vi "Interfaz grafica - corriente.vi"() -> ()   [LabVIEW 2024]
uses:
  160620 Optotune Lens Driver 4 Labview package/Hello Optotune Lens (30.06.2015)/Calibration.ctl
  <vilib>/DAQmx/read.llb/DAQmx Read (Analog 1D Wfm NChan NSamp).vi
  <vilib>/Analysis/2dsp.llb/Decimate (single shot, DBL).vi
  <vilib>/Utility/file.llb/Read Delimited Spreadsheet (string).vi
  <vilib>/Instr/_visa.llb/VISA Configure Serial Port (Instr).vi
  <vilib>/DAQmx/create/channels.llb/DAQmx Create Channel (AI-Voltage-Basic).vi
  <vilib>/DAQmx/configure/timing.llb/DAQmx Timing (Sample Clock).vi
  <vilib>/DAQmx/miscellaneous.llb/DAQmx Fill In Error Info.vi
  <vilib>/Waveform/WDTOps.llb/WDT Index Channel DBL.vi
  <vilib>/Analysis/2dsp.llb/Decimate (continuous, DBL).vi
  <vilib>/Utility/file.llb/Write Delimited Spreadsheet (string).vi
  <vilib>/Waveform/WDTOps.llb/WDT Get Waveform Time Array DBL.vi
  <vilib>/Analysis/NI_AALPro.lvlib
panel:
  out "Array 4":string[](array[string])
  out "Array 3":string[](array[string])
  out "Array 2":string[](array[string])
  out "Array":string[](array[string])
  out "Nombre 2":string
  in  "Restablecer Iniciales":bool
  in  "Incremento":dbl=0.1 format="%#_13g"
  out "Potencia derecho":dbl
  out "error out 4":errorcluster
  out "error out 3":errorcluster
  out "error out 2":errorcluster
  in  "Tab Control 3":enum32{"WL", "Video"}(tab)
  out "Waveform length":dbl[][](graph)
  in  "Minimo escala Y":dbl format="%#_13g"
  in  "Maximo escala Y":dbl format="%#_13g"
  in  "Escala autom. Y":u8=1
  in  "Escala autom. X":u8=1
  in  "Maximo escala X":dbl
  in  "Minimo escala X":dbl
  out "Image Out":T1(plugin-control)
  in  "Frame Rate":u32=30
  in  "Modo de video":u16(ring)=21 items=["160x90 I420 30 fps", "160x90 MJPG 30 fps", "160x90 RGB24 30 fps", "160x120 I420 30 fps", "160x120 MJPG 30 fps", "160x120 RGB24 30 fps", "176x144 I420 30 fps", "176x144 MJPG 30 fps", "176x144 RGB24 30 fps", "320x180 I420 30 fps", "320x180 MJPG 30 fps", "320x180 RGB24 30 fps", "320x240  I420 30 fps", "320x240 MJPG 30 fps", "320x240 RGB24 30 fps", "352x288 I420 30 fps", "352x288 MJPG 30 fps", "352x288 RGB24 30 fps", "432x240 I420 30 fps", "432x240 MJPG 30 fps", "432x240 RGB24 30 fps", "640x360 I420 30 fps", "640x360 MJPG 30 fps", "640x360 RGB24 30 fps", "640x480 I420 30 fps", "640x480 MJPG 30 fps", "640x480 RGB24 30 fps", "800x448 I420 30 fps", "800x448 MJPG 30 fps", "800x448 RGB24 30 fps", "800x600 I420 30 fps", "800x600 MJPG 30 fps", "800x600 RGB24 30 fps", "864x480 I420 30 fps", "864x480 MJPG 30 fps", "864x480 RGB24 30 fps", "960x720 I420 30 fps", "960x720 MJPG 30 fps", "960x720 RGB24 30 fps", "1024x576 I420 30 fps", "1024x576 MJPG 30 fps", "1024x576 RGB24 30 fps", "1280x720 I420 30 fps", "1280x720 MJPG 30 fps", "1280x720 RGB24 30 fps", "1600x896 I420 30 fps", "1600x896 MJPG 30 fps", "1600x896 RGB24 30 fps", "1920x1080 I420 5 fps", "1920x1080 MJPG 30 fps", "1920x1080 RGB24 5 fps", "2304x1296 I420 2 fps", "2304x1296 RGB24 2 fps", "2304x1536 I420 2 fps", "2304x1536 RGB24 2 fps"]
  in  "Carpeta archivo":string="C:\\Users\\TGM1603\\Documents\\LabVIEW Data\\Experimentos electrodos\\VideosExperimentos"
  in  "Calidad":u32=1000
  out "VISA resource name out":string
  in  "Tab Control 2":T2(tab)
  in  "DAQmx Physical Channel":tag
  in  "Frecuencia muestreo":i32=20000
  in  "tamaño buffer":i32=1000
  in  "factor decimacion":i32=20
  in  "Ganancia":u16(ring) items=["0.2"=51455, "1"=33023, "10"=49407, "20"=41215, "30"=57599, "40"=37119, "60"=53503, "80"=45311, "120"=61695, "157"=35071, ""=0]
  in  "Potencia inicial lente derecho":dbl(slide) scale=-3.0..3.0
  in  "Potencia inicial lente izquierdo":dbl(slide) scale=-3.0..3.0
  in  "VISA resource name":string="COM11"
  in  "VISA resource name 2":string="COM10"
  out "DPT INICIALES D":dbl
  out "DPT INICIALES I":dbl
  out "Potencia izquierdo":dbl
  in  "error in (no error) 5":errorcluster
  in  "error in (no error) 4":errorcluster
  in  "error in (no error) 3":errorcluster
  in  "error in (no error) 2":errorcluster
  in  "Calibration 4":T3={"Max Current A"=293.0, "Max Current B"=293.0, "UCL A"=300.0, "UCL B"=300.0, "LCL A"=0.0, "LCL B"=0.0} {"Max Current A" format="%#_g mA"; "Max Current B" format="%#_g mA"; "UCL A" format="%#_g mA"; "LCL A" format="%#_g mA"; "UCL B" format="%#_g mA"; "LCL B" format="%#_g mA"}
  out "ID 2":u16
  out "VISA resource name out 2":string
  out "Calibration 3":T3 {"Max Current A" format="%#_g mA"; "Max Current B" format="%#_g mA"; "UCL A" format="%#_g mA"; "LCL A" format="%#_g mA"; "UCL B" format="%#_g mA"; "LCL B" format="%#_g mA"}
  out "OK 2":bool
  out "Data 2":string
  out "Command to Port 2":string
  in  "Cola tipo 2":dbl[](array[numeric])
  out "Distancia":u32
  in  "Tamaño ventana WL":i32=60
  in  "Limite inferior WL":dbl=25.0 format="%#_13g"
  in  "Limite superior WL":dbl=50.0
  out "number":u32
  in  "Calibration":T3={"Max Current A"=293.0, "Max Current B"=293.0, "UCL A"=300.0, "UCL B"=300.0, "LCL A"=0.0, "LCL B"=0.0} {"Max Current A" format="%#_g mA"; "Max Current B" format="%#_g mA"; "UCL A" format="%#_g mA"; "LCL A" format="%#_g mA"; "UCL B" format="%#_g mA"; "LCL B" format="%#_g mA"}
  out "ID":u16
  out "Calibration 2":T3 {"Max Current A" format="%#_g mA"; "Max Current B" format="%#_g mA"; "UCL A" format="%#_g mA"; "LCL A" format="%#_g mA"; "UCL B" format="%#_g mA"; "LCL B" format="%#_g mA"}
  out "OK":bool
  out "Data":string
  out "Command to Port":string
  in  "DPT dif.":dbl
  out "error out":errorcluster
  in  "error in (no error)":errorcluster
  in  "WL":dbl
  in  "Cola tipo":dbl[](array[numeric])
  out "T button?":bool
  in  "Elegir menu Exp":bool
  in  "Elegir menu":bool
  out "path":path
  in  "Iniciar experimento":bool
  in  "Parar adquisicion":bool
  out "Enfermedad visual":string
  out "Edad":string
  out "Nombre":string
  out "Cedula":string
  in  "Carpeta":path=path "C:/Users/TGM1603/Documents/LabVIEW Data/Experimentos electrodos"
  in  "?":bool
  in  "Menu Principal":u16(ring) items=["Visualizacion general ", "Llevar a cabo un experimento", "Ajustar potencia inicial lentes"]
  in  "Menu experimentos":u16(ring) items=["Experimento 1", "Experimento 2", "Experimento 3", "Experimento 4"]
  in  "Tab Control":enum32{"Señal EMG", "Potencia y distancia"}(tab)
  out "Senal EMG":waveform(dbl)[](graph)
  in  "Escala automatica Y":u8
  in  "Escala automatica X":u8=1
  in  "X Scale.Range:Increment":dbl
  in  "X Scale.Range:Minimum":dbl
  in  "X Scale.Range:Maximum":dbl
  in  "Y Scale.Range:Minimum":dbl=-5.0
  in  "Y Scale.Range:Maximum":dbl=5.0
  in  "Escala Y min":dbl
  in  "Escala Y max":dbl
  in  "Auto scale Y":u8=1
  in  "Escala X max":dbl
  in  "Escala X min":dbl
  out "Potencia optica y distancia":dbl[][](graph)
  in  "Auto scale X":u8=1
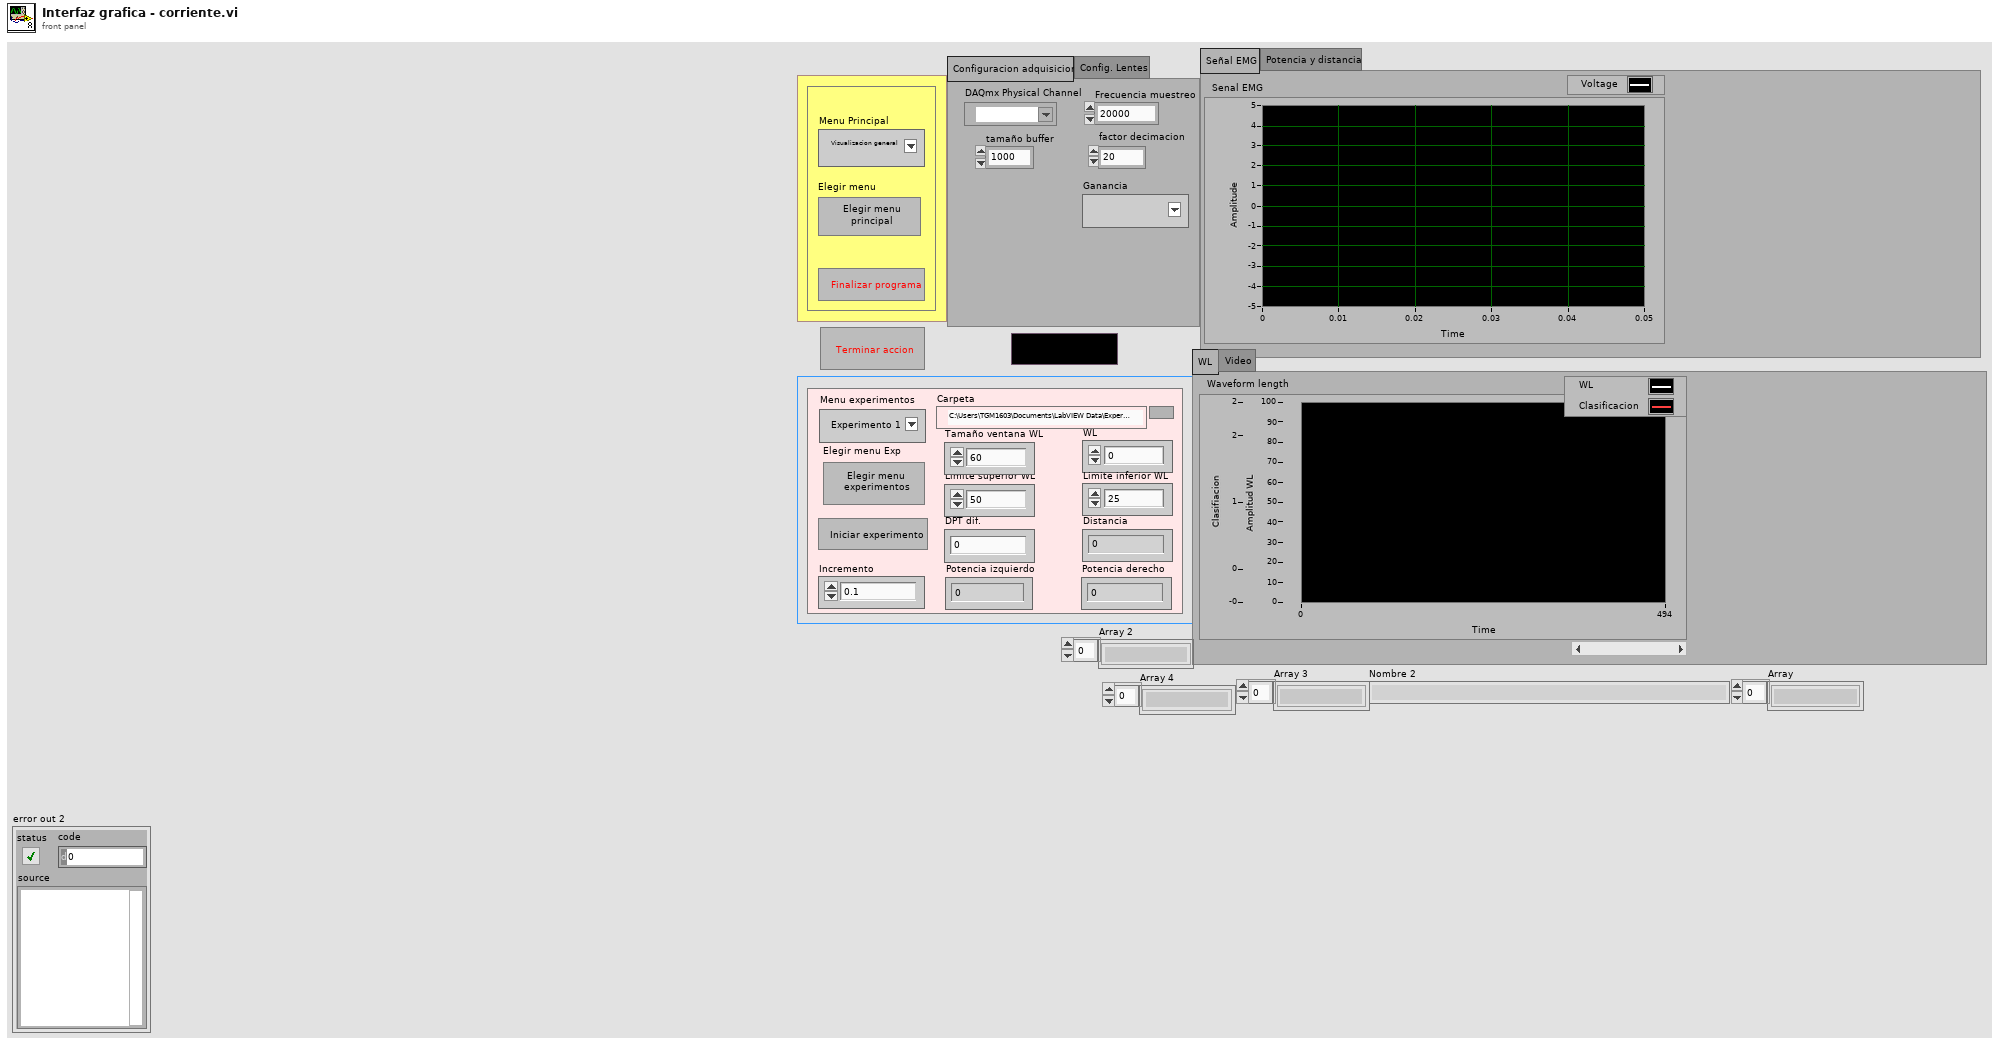
[diagram p1: front panel]
types:
  T1 = typedef "IMAQ Image.ctl" = refnum<image>
  T2 = enum32{"Configuracion adquisicion", "Config. Lentes"}
  T3 = typedef "Calibration.ctl" = cluster{"Max Current A":dbl, "Max Current B":dbl, "UCL A":dbl, "UCL B":dbl, "LCL A":dbl, "LCL B":dbl}
  T4 = enum16{"Left Button", "Center Button", "Right Button", "Window Close"}
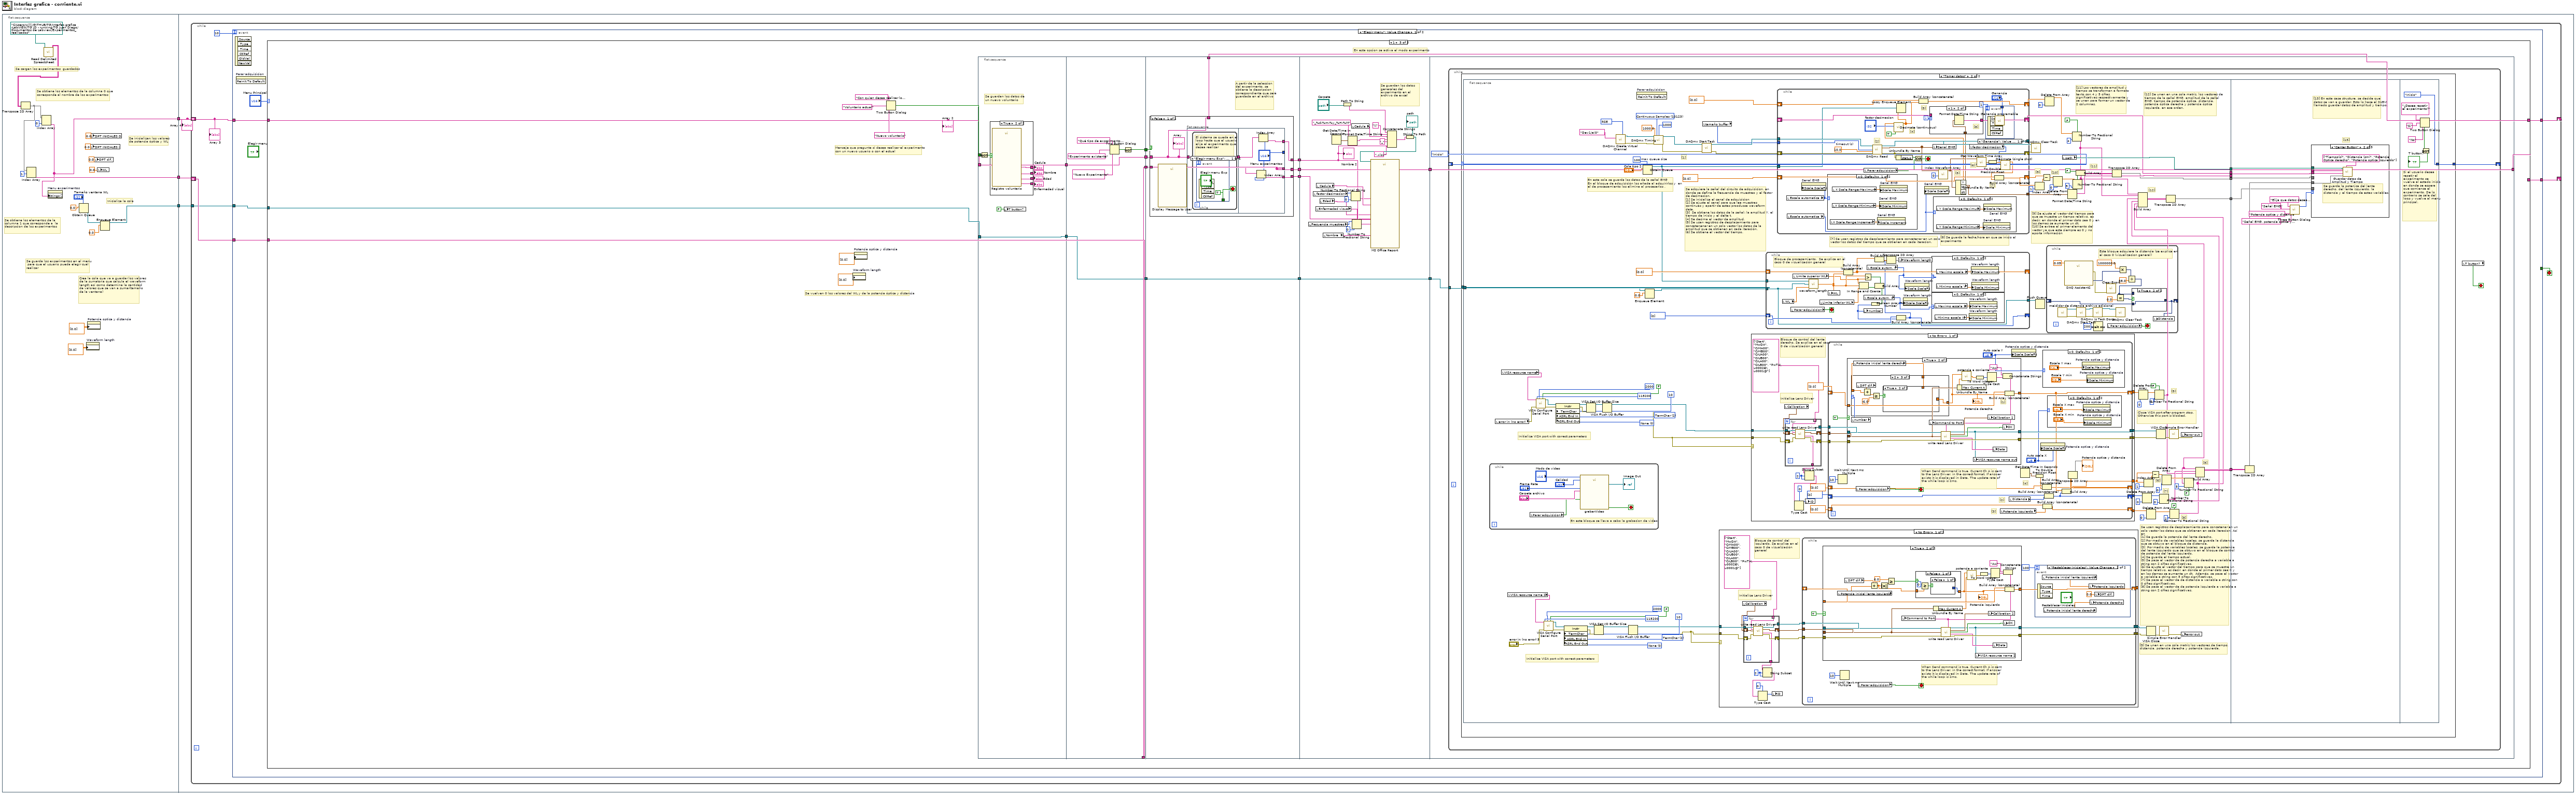
[diagram p0: block diagram]
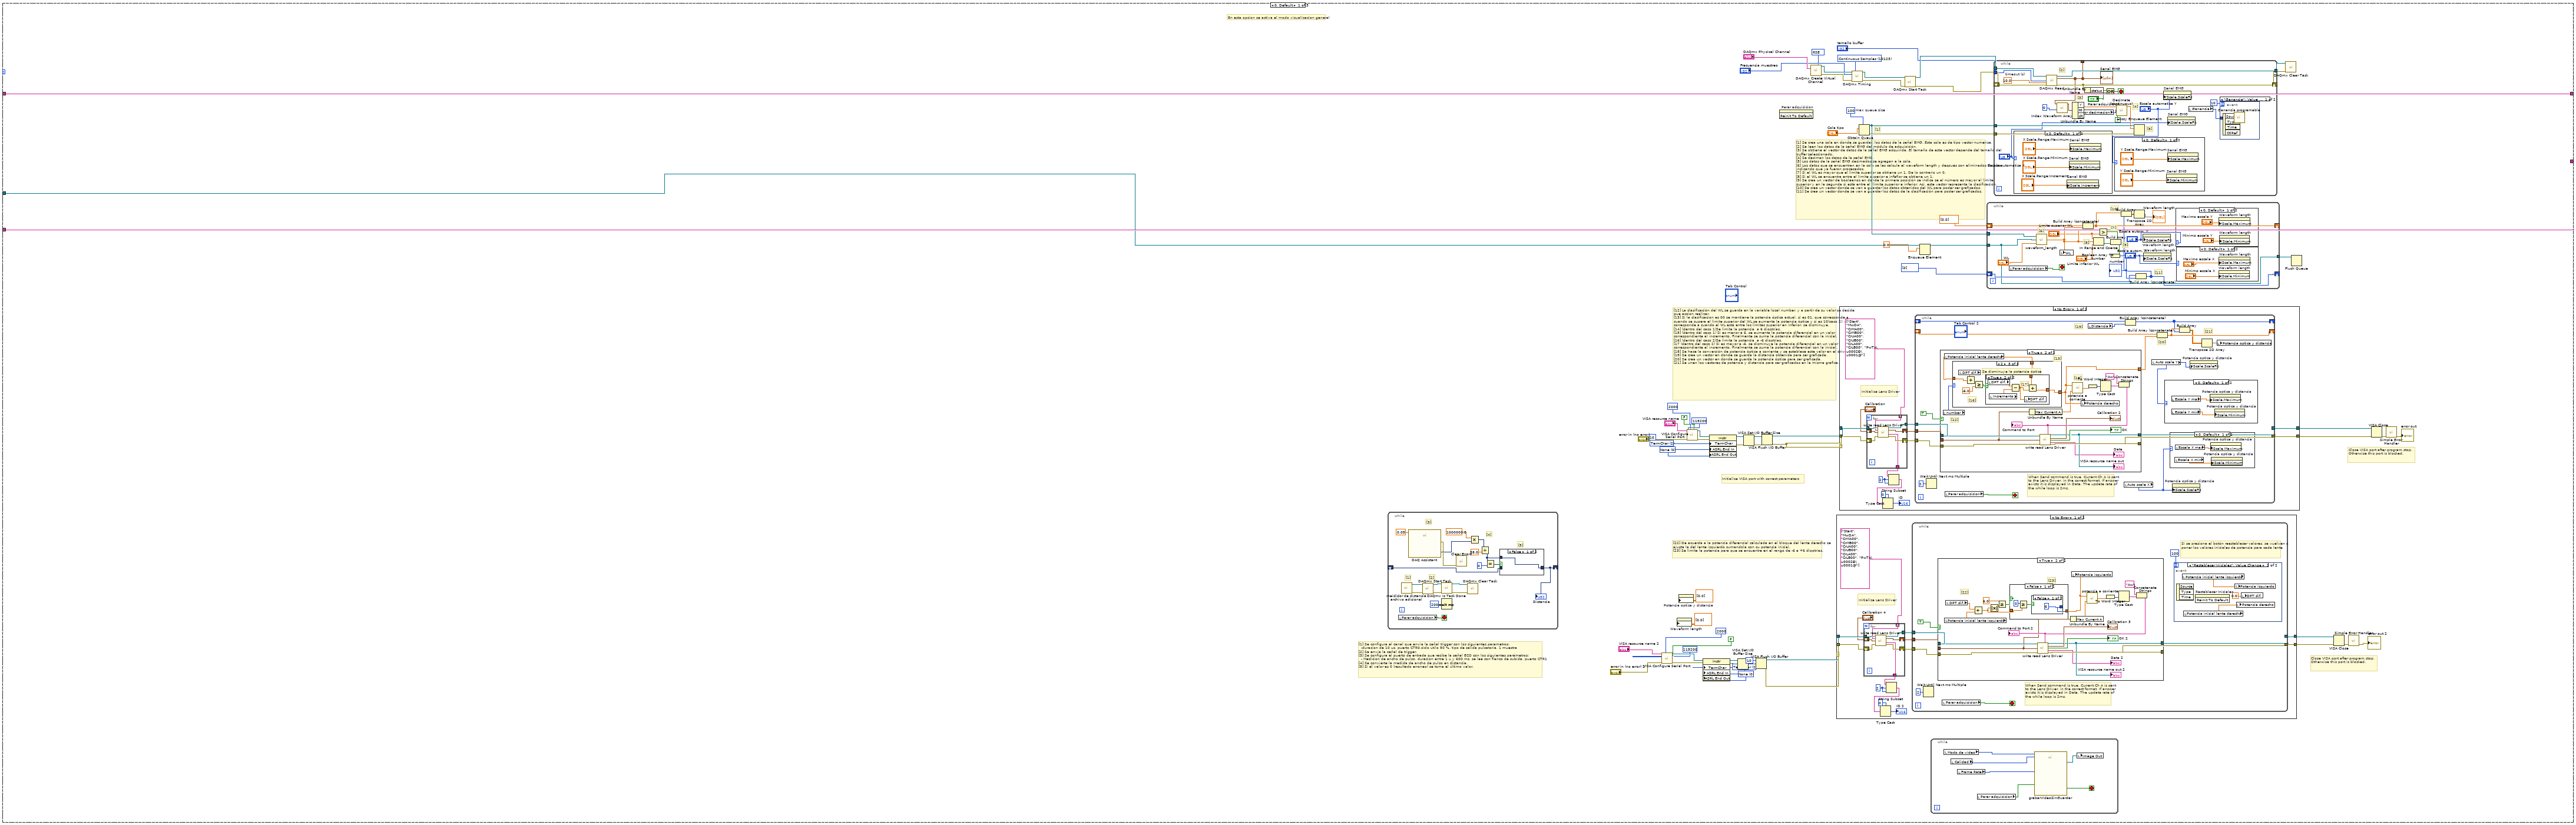
[diagram p2: hidden frame]
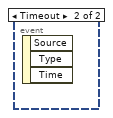
[diagram p3: hidden frame]
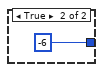
[diagram p5: hidden frame]
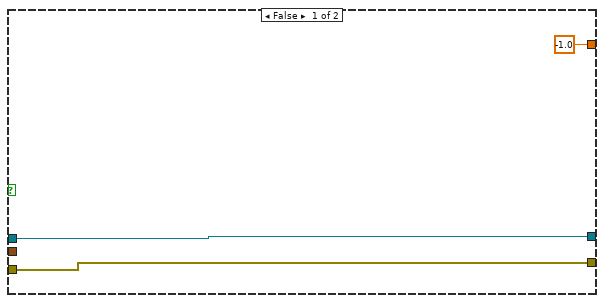
[diagram p11: hidden frame]
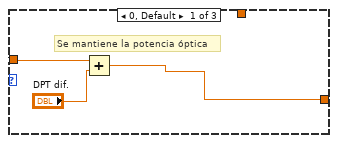
[diagram p12: hidden frame]
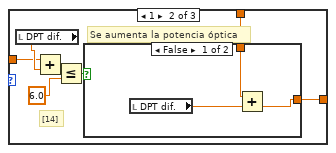
[diagram p13: hidden frame]
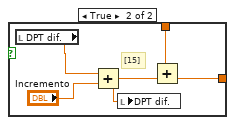
[diagram p14: hidden frame]
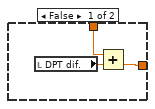
[diagram p15: hidden frame]
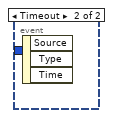
[diagram p19: hidden frame]
diagram:
  n1 = flat-sequence {
    tunnel: [w18] -> w3
    tunnel: [w15] -> w2
    tunnel: [w10] -> w1
    tunnel: w3 -> [w22]
    tunnel: w2 -> [w24]
    tunnel: w1 -> [w23]
    frame #0 {
      # "Se inicializan los valores\nde potencia óptica y WL"
      # "Inicializa la cola"
      # "Crea la cola que va a guardar los valores de la sumatoria que calcula el waveform length así como determina la cantidad de valores que se van a sumar(tamaño de la ventana)"
      # "Se obtiene los elementos de la columna 1 que corresponde a  la descripcion de los experimentos"
      # "Se obtiene los elementos de la columna 0 que corresponde al nombre de los experimentos"
      # "Se guarda los experimentos en el menu\n para que el usuario pueda elegir cual \nrealizar"
      # "Se cargan los experimentos  guardados"
      n2 = call-poly <vilib>:"Read Delimited Spreadsheet.vi"("file path (dialog if empty)"=path "C:/Users/willi/GITHUB/TG/Interfaz grafica -LabVIEW/TG JD - running/TG Juan Diego/Documentos de Labview/Experimentos_realizados") -> ("all rows"=w19:string[][])  [unwired: 9 in, 5 out]
      n3 = Transpose 2D Array(2D array=w19) -> (transposed array=w16:string[][])
      n4 = Index Array(array=w16, index (row)=1) -> (element=w15:string[])  [unwired: 1 in]
      n5 = Index Array(array=w16, index (row)=0) -> (element=w18:string[])  [unwired: 1 in]
      n6 = property on="Menu experimentos" class="Ring (strict)"("Strings []"=w18) -> ()  [unwired: 2 in, 2 out]
      n7 = Obtain Queue(max queue size (-1, unlimited)="Tamaño ventana WL", element data type=0.0) -> (queue out=w13:refnum<queue>)  [unwired: 3 in, 2 out]
      n8 = property on="Waveform length" class="WFChart (strict)"("History Data"=dbl[][] [[0.0]]) -> ()  [unwired: 2 in, 2 out]
      n9 = property on="Potencia optica y distancia" class="WFChart (strict)"("History Data"=dbl[][] [[0.0]]) -> ()  [unwired: 2 in, 2 out]
      n10 = local write "DPT INICIALES D"(0.0 ("DPT INIT.1")) -> ()
      n11 = local write "DPT INICIALES I"(0.0 ("DPT INIT.2")) -> ()
      n12 = local write "DPT dif."(0.0 ("WL")) -> ()
      n13 = local write "WL"(0.0 ("WL")) -> ()
      n14 = Enqueue Element(queue=w13, element=0.0) -> (queue out=w10:refnum<queue>)  [unwired: 2 in, 2 out]
    }
    frame #1 {
      n15 = while {
        shift-right: [w30] -> _
        shift-left: w22 -> [w31]
        shift-right: [w28] -> _
        shift-left: w24 -> [w29]
        tunnel: w23 -> [w27]
        stop <- w26 stop-if-true
        n16 = event shown="[0] \"Elegir menu\": Value Change" {
          selector: _ -> [_ _]
          dyn-events: _ -> [_ _]
          timeout: 10 -> [_ _]
          tunnel: w31 -> [w37 w1052]
          tunnel: [w36 w1052] -> w30
          tunnel: w29 -> [w35 w1051]
          tunnel: [w34 w1051] -> w28
          tunnel: w27 -> [w32 _]
          tunnel: [_ "?"] -> w26
          event "Elegir menu": Value Change {
            n17 = event-data() -> ()  [unwired: 1 in, 6 out]
            n18 = invoke on="Parar adquisicion" class="Bool (strict)" method="Reinit To Default"() -> ()  [unwired: 3 in, 3 out]
            n19 = case shown="1" "Menu Principal" {
              tunnel: w37 -> [w104 w389 w509]
              tunnel: [w104 w389 w508] -> w36
              tunnel: w35 -> [w103 w388 w506]
              tunnel: [w103 w388 w505] -> w34
              tunnel: w32 -> [w93 _ w496]
              frame 0, Default {
                w38 = 10123 items=["Finite Samples"=10178, "Continuous Samples"=10123, "Hardware Timed Single Point"=12522] ("sample mode")
                w39 = 10083 items=["Default"=-1, "RSE"=10083, "NRSE"=10078, "Differential"=10106, "Pseudodifferential"=12529] ("input terminal configuration")
                w61 = u16 0 items=["None", "Last Bit", "TermChar", "Break"] ("Serial Settings:End Mode for Writes")
                w60 = u16 2 items=["None", "Last Bit", "TermChar"] ("Serial Settings:End Mode for Reads")
                w83 = u16 0 items=["None", "Last Bit", "TermChar", "Break"] ("Serial Settings:End Mode for Writes")
                w84 = u16 2 items=["None", "Last Bit", "TermChar"] ("Serial Settings:End Mode for Reads")
                w97 = 100  # max queue size
                # "[22] De acuerda a la potencia diferencial calculada en el bloque del lente derecho se ajusta la del lente izquierdo sumandola con su potencia inicial.\n[23] Se limita la potencia para que se encuentre en el rango de -6 a +6 dioptrías."
                # "[12] La clasificación del WL se guarda en la variable local number, y a partir de su valor se decide que accion realizar.\n[13] Si la clasificacion es 00 se mantiene la potencia óptica actual, si es 01, que corresponde a cuando se supera el limite superior del WL,se aumenta la potencia óptica y si es 10(caso 2), que corresponde a cuando el WL está entre los limites superior en inferior, se disminuye. \n[14] (dentro del caso 1)Se limita la potencia  a 6 dioptrías. \n[15] (dentro del caso 1) Si es menor a 6, se aumenta la potencia diferencial en un valor correspondiente al incremento. Finalmente se suma la potencia diferencial con la inicial.\n[16] (dentro del caso 2)Se limita la potencia  a -6 dioptrías.\n[17 (dentro del caso 2) Si es mayor a -6, se disminuye la potencia diferencial en un valor correspondiente al incremento. Finalmente se suma la potencia diferencial con la inicial.\n[18] Se hace la conversión de potencia óptica a corriente y se establece este valor en el driver.\n[19] Se crea un vector en donde se guarda la distancia obtenida para ser graficada.\n[20] Se crea un vector en donde se guarda la potencia óptica para ser graficada.\n[21] Se unen los vectores de potencia y distancia para ser graficados en la misma grafica."
                # "[1] Se crea una cola en donde se guardan los datos de la señal EMG. Esta cola es de tipo vector numerica.\n[2] Se leen los datos de la señal EMG del módulo de adquisición. \n[3] Se obtiene el vector de datos de la señal EMG adquirida. El tamaño de este vector depende del tamaño del buffer seleccionado.\n[4] Se deciman los datos de la señal EMG.\n[5] Los datos de la señal EMG decimados se agregan a la cola.\n[6] Los datos que se encuentran en la cola se les calcula el waveform length y después son eliminados de esta, indicando que ya fueron procesados. \n[7] Si el WL es mayor que el limite superior se obtiene un 1. De lo contrario un 0.\n[8] Si el WL se encuentra entre el límite superior e infefior se obtiene un 1.\n[9] Se crea un vector de booleanos en donde la primera posición se indica se el número es mayor al límite superior y en la segunda si está entre el  limite superior e inferior. Así, este vector representa la clasificación.\n[10] Se crea un vector donde se van a guardar los datos obtenidos del WL para poder ser graficados.\n[11] Se crea un vector donde se van a guardar los datos de la clasificación para poder ser graficados."
                # "[1]"
                # "En esta opcion se activa el modo visualizacion general"
                # "Close VISA port after program stop. Otherwise this port is blocked."
                # "[1] Se configura el canal que envía la señal trigger con los siguientes parametros:\n  -duracion de 10 us, puerto CTR0,ciclo utilo 50 %, tipo de salida pulsatoria, 1 muestra \n[2] Se envía la señal de trigger.\n[3] Se configura el puerto de entrada que recibe la señal ECO con los siguientes parámetros:\n  - Medicion de ancho de pulso, duracion entre 1 u y 600 ms, se lee con flanco de subida, puerto CTR1\n[4] Se convierte la medida de ancho de pulso en distancia.\n[5] Si el valor es 0 (resultado erroneo) se toma el último valor."
                # "Close VISA port after program stop. Otherwise this port is blocked."
                # "Initialize VISA port with correct parameters"
                n20 = while {
                  shift-right: [w178] -> _
                  shift-left: _ -> [w177]
                  stop <- w182 stop-if-true
                  # "[5]"
                  # "[4]"
                  # "[3]"
                  # "[2]"
                  # "[1]"
                  n21 = local read "Parar adquisicion"() -> (w182:bool)
                  n22 = call "meididor de distancia archivo adicional.vi"() -> ("error out"=w185:errorcluster, "task out"=w186:refnum<k21>)  [unwired: 10 in]
                  n23 = call "DAQ Assistant"("timeout (s)"=0.05) -> ("data"=w195:dynamicdata, "error out"=w183:errorcluster)  [unwired: 16 in, 1 out]
                  n24 = call <vilib>:"DAQmx Start Task.vi"("task/channels in"=w186, "error in"=w185) -> ("task out"=w189:refnum<k21>, "error out"=w190:errorcluster)  [unwired: 12 in]
                  n25 = call <vilib>:"DAQmx Is Task Done.vi"("task/channels in"=w189, "error in"=w190) -> ("task out"=w187:refnum<k21>, "error out"=w188:errorcluster)  [unwired: 11 in, 1 out]
                  n26 = Wait (ms)(milliseconds to wait=u32 200) -> ()  [unwired: 1 out]
                  n27 = call <vilib>:"Clear Errors.vi"("error in (no error)"=w183) -> ()  [unwired: 5 in, 2 out]
                  n28 = call <vilib>:"DAQmx Clear Task.vi"("task in"=w187, "error in"=w188) -> ()  [unwired: 13 in, 1 out]
                  n29 = Multiply(x=1000000.0, y=w195) -> (x*y=w193:dynamicdata)
                  n30 = Divide(x=w193, y=58.0) -> (x/y=w179:dynamicdata)
                  n31 = Equal?(x=w179, y=u16 0) -> (x = y?=w181:dynamicdata)
                  n32 = case shown="False" w181 {
                    tunnel: [w196 w197] -> w178
                    tunnel: w179 -> [w196 _]
                    tunnel: w177 -> [_ w197]
                    frame False {
                    }
                    frame True {
                    }
                  }
                  "Distancia" <- w178
                }
                n33 = call-poly "VISA Configure Serial Port"("VISA resource name"="VISA resource name 2", "timeout (10sec)"=u32 2000, "Enable Termination\nChar (T)"=FALSE ("Enable Termination\nChar (T)"), "baud rate (9600)"=u32 115200, "error in (no error)"="error in (no error) 2") -> ("VISA resource name out"=w56:refnum<visa-resource-name>, "error out"=w58:errorcluster)  [unwired: 9 in]
                n34 = property on="Waveform length" class="WFChart (strict)"("History Data"=dbl[][] [[0.0]]) -> ()  [unwired: 2 in, 2 out]
                n35 = property on="Potencia optica y distancia" class="WFChart (strict)"("History Data"=dbl[][] [[0.0]]) -> ()  [unwired: 2 in, 2 out]
                n36 = call-poly "VISA Configure Serial Port"("VISA resource name"="VISA resource name", "timeout (10sec)"=u32 2000, "Enable Termination\nChar (T)"=FALSE ("Enable Termination\nChar (T)"), "baud rate (9600)"=u32 115200, "error in (no error)"="error in (no error)") -> ("VISA resource name out"=w88:refnum<visa-resource-name>, "error out"=w86:errorcluster)  [unwired: 9 in]
                n37 = property class="Instr"(reference=w56, error in=w58, "TermChar"=u8 10 ("Message Based Settings:Termination Character"), "ASRL End In"=w60, "ASRL End Out"=w61) -> (reference out=w57:refnum<visa-resource-name>, error out=w59:errorcluster)
                n38 = property class="Instr"(reference=w88, error in=w86, "TermChar"=u8 10 ("Message Based Settings:Termination Character"), "ASRL End In"=w84, "ASRL End Out"=w83) -> (reference out=w87:refnum<visa-resource-name>, error out=w85:errorcluster)
                n39 = VISA Set I/O Buffer Size(VISA resource name=w57, error in (no error)=w59) -> (VISA resource name out=w64:refnum<visa-resource-name>, error out=w65:errorcluster)  [unwired: 2 in]
                n40 = VISA Set I/O Buffer Size(VISA resource name=w87, error in (no error)=w85) -> (VISA resource name out=w80:refnum<visa-resource-name>, error out=w79:errorcluster)  [unwired: 2 in]
                n41 = VISA Flush I/O Buffer(VISA resource name=w64, error in (no error)=w65) -> (VISA resource name out=w50:refnum<visa-resource-name>, error out=w51:errorcluster)  [unwired: 1 in]
                n42 = VISA Flush I/O Buffer(VISA resource name=w80, error in (no error)=w79) -> (VISA resource name out=w78:refnum<visa-resource-name>, error out=w73:errorcluster)  [unwired: 1 in]
                n43 = invoke on="Parar adquisicion" class="Bool (strict)" method="Reinit To Default"() -> ()  [unwired: 3 in, 3 out]
                n44 = call-poly <vilib>:"DAQmx Create Virtual Channel.vi"("input terminal configuration"=w39, "physical channels"="DAQmx Physical Channel") -> ("task out"=w45:refnum<k21>, "error out"=w44:errorcluster)  [unwired: 12 in]
                n45 = case shown="No Error" w51 {
                  tunnel: w51 -> [w124 w175]
                  tunnel: w50 -> [w123 w176]
                  tunnel: [w122 w175] -> w46
                  tunnel: [w121 w176] -> w47
                  frame No Error {
                    w119 = 2 ("length (rest)")
                    # "Initialize Lens Driver"
                    n46 = for {
                      tunnel: w123 -> [w173]
                      tunnel: [w170] -> w113
                      tunnel: string[] ["Start", "MwDA", "CrMA00", "CrMB00", "CrUA00", "CrUB00", "CrLA00", "CrLB00", "PwTA\u0002Ð\u0001@"] -> [w168] mode=indexing
                      tunnel: [w167] -> w112
                      shift-right: [w171] -> w114
                      shift-left: "Calibration 4" -> [w172]
                      shift-right: [w169] -> w115
                      shift-left: w124 -> [w174]
                      n47 = call "write read Lens Driver.vi"("VISA resource name"=w173, "command"=w168, "Calibration"=w172, "error in (no error)"=w174) -> ("VISA resource name out"=w170:refnum<visa-resource-name>, "Calibration 2"=w171:T3, "Data"=w167:string, "error out"=w169:errorcluster)  [unwired: 4 in, 4 out]
                    }
                    n48 = String Subset(string=w112, offset (0)=w119, length (rest)=w119) -> (substring=w117:string)
                    n49 = Type Cast(type=u16 0 ("length (rest)"), x=w117) -> (*(type *) &x=→"ID 2":u16)
                    n50 = while {
                      tunnel: [w127] -> w122
                      tunnel: [w128] -> w121
                      tunnel: w115 -> [w133]
                      tunnel: w114 -> [w132]
                      tunnel: w113 -> [w131]
                      stop <- w126 stop-if-true
                      # "Si se presiona el botón reestablecer valores, se vuelven a poner los valores iniciales de potencia para cada lente"
                      # "When Send command is true, Current Ch A is sent to the Lens Driver, in the correct format. If answer exists it is displayed in Data. The update rate of the while loop is 2ms."
                      n51 = Wait Until Next ms Multiple(millisecond multiple=u32 2) -> ()  [unwired: 1 out]
                      n52 = case shown="True" TRUE ("Send command") {
                        tunnel: [w138 w159] -> w127
                        tunnel: w133 -> [w138 w158]
                        tunnel: w132 -> [_ w140]
                        tunnel: w131 -> [w137 w157]
                        tunnel: [w137 w154] -> w128
                        frame False {
                        }
                        frame True {
                          # "[23]"
                          # "[22]"
                          n53 = local read "Potencia inicial lente izquierdo"() -> (w148:dbl)
                          n54 = local read "DPT dif."() -> (w149:dbl)
                          n55 = Add(x=w149, y=w148) -> (x+y=w144:dbl)
                          n56 = Absolute Value(x=w144) -> (abs(x)=w146:dbl)
                          n57 = Greater Or Equal?(x=6.0, y=w146) -> (x >= y?=w147:bool)
                          n58 = case shown="False" w147 {
                            tunnel: w144 -> [w162 w166]
                            tunnel: [w160 w166] -> w142
                            frame False {
                              n59 = Greater Or Equal?(x=u16 0, y=w162) -> (x >= y?=w163:bool)
                              n60 = case shown="False" w163 {
                                tunnel: [i16 6 ("x") i16 -6 ("x")] -> w160
                                frame False {
                                }
                                frame True {
                                }
                              }
                            }
                            frame True {
                            }
                          }
                          n61 = Unbundle By Name(w140) -> ("Max Current A"=w141:dbl)
                          n62 = local write "Potencia izquierdo"(w142) -> ()
                          n63 = call "potencia a corriente.vi"("Max current A"=w141, "Potencia"=w142) -> ("Corriente"=w143:dbl)
                          n64 = To Word Integer(number=w143) -> (16bit integer=w152:i16)
                          n65 = Type Cast(x=w152) -> (*(type *) &x=w151:string)  [unwired: 1 in]
                          n66 = Concatenate Strings("Aw", w151) -> (w150:string)
                          "Command to Port 2" <- w150
                          n67 = call "write read Lens Driver.vi"("VISA resource name"=w157, "command"=w150, "Calibration"=w140, "error in (no error)"=w158) -> ("VISA resource name out"=w154:refnum<visa-resource-name>, "Calibration 2"=→"Calibration 3":T3, "OK"=→"OK 2":bool, "Data"=→"Data 2":string, "error out"=w159:errorcluster)  [unwired: 4 in, 3 out]
                          "VISA resource name out 2" <- w154
                        }
                      }
                      n68 = local read "Parar adquisicion"() -> (w126:bool)
                      n69 = event shown="[0] \"Restablecer Iniciales\": Value Change" {
                        selector: _ -> [_ _]
                        dyn-events: _ -> [_ _]
                        timeout: 100 -> [_ _]
                        event "Restablecer Iniciales": Value Change {
                          n70 = event-data() -> ()  [unwired: 1 in, 3 out]
                          n71 = local read "Potencia inicial lente izquierdo"() -> (w134:dbl)
                          n72 = local read "Potencia inicial lente derecho"() -> (w135:dbl)
                          n73 = invoke on="Restablecer Iniciales" class="Bool" method="Reinit To Default"() -> ()  [unwired: 3 in, 3 out]
                          n74 = local write "Potencia izquierdo"(w134) -> ()
                          n75 = local write "Potencia derecho"(w135) -> ()
                          n76 = local write "DPT dif."(0.0 ("DPT dif.")) -> ()
                        }
                        event Timeout {
                          n77 = event-data() -> ()  [unwired: 1 in, 3 out]
                        }
                      }
                    }
                  }
                  frame Error {
                  }
                }
                n78 = case shown="No Error" w73 {
                  tunnel: w73 -> [w211 w295]
                  tunnel: w78 -> [w210 w296]
                  tunnel: [w209 w295] -> w76
                  tunnel: [w208 w296] -> w74
                  frame No Error {
                    w206 = 2 ("length (rest)")
                    # "Initialize Lens Driver"
                    n79 = for {
                      tunnel: w210 -> [w293]
                      tunnel: [w290] -> w200
                      tunnel: string[] ["Start", "MwDA", "CrMA00", "CrMB00", "CrUA00", "CrUB00", "CrLA00", "CrLB00", "PwTA\u0002Ð\u0001@"] -> [w288] mode=indexing
                      tunnel: [w287] -> w199
                      shift-right: [w291] -> w201
                      shift-left: "Calibration" -> [w292]
                      shift-right: [w289] -> w202
                      shift-left: w211 -> [w294]
                      n80 = call "write read Lens Driver.vi"("VISA resource name"=w293, "command"=w288, "Calibration"=w292, "error in (no error)"=w294) -> ("VISA resource name out"=w290:refnum<visa-resource-name>, "Calibration 2"=w291:T3, "Data"=w287:string, "error out"=w289:errorcluster)  [unwired: 4 in, 4 out]
                    }
                    n81 = String Subset(string=w199, offset (0)=w206, length (rest)=w206) -> (substring=w204:string)
                    n82 = Type Cast(type=u16 0 ("length (rest)"), x=w204) -> (*(type *) &x=→"ID":u16)
                    n83 = while {
                      tunnel: [w223] -> w209
                      tunnel: [w224] -> w208
                      tunnel: w202 -> [w229]
                      tunnel: w201 -> [w228]
                      tunnel: w200 -> [w227]
                      shift-right: [w214] -> _
                      shift-left: _ -> [w218]
                      shift-right: [w215] -> _
                      shift-left: _ -> [w217]
                      stop <- w222 stop-if-true
                      # "[21]"
                      # "[20]"
                      # "[19]"
                      # "When Send command is true, Current Ch A is sent to the Lens Driver, in the correct format. If answer exists it is displayed in Data. The update rate of the while loop is 2ms."
                      n84 = Wait Until Next ms Multiple(millisecond multiple=u32 2) -> ()  [unwired: 1 out]
                      n85 = case shown="True" TRUE ("Send command") {
                        tunnel: [w236 w253] -> w223
                        tunnel: w229 -> [w236 w252]
                        tunnel: w228 -> [_ w239]
                        tunnel: w227 -> [w235 w251]
                        tunnel: [w235 w248] -> w224
                        tunnel: [-1.0 ("DPT") w241] -> w216
                        frame False {
                        }
                        frame True {
                          # "[18]"
                          # "[13]"
                          # "[12]"
                          n86 = local read "number"() -> (w243:u32)
                          n87 = local read "Potencia inicial lente derecho"() -> (w242:dbl)
                          n88 = case shown="2" w243 {
                            tunnel: [w255 w263 w278] -> w241
                            tunnel: w242 -> [w256 w258 w273]
                            tunnel: w242 -> [_ w257 w272]
                            frame 0, Default {
                              # "Se mantiene la potencia óptica"
                              n89 = Add(x=w256, y="DPT dif.") -> (x+y=w255:dbl)
                            }
                            frame 1 {
                              # "[14]"
                              # "Se aumenta la potencia óptica"
                              n90 = local read "DPT dif."() -> (w259:dbl)
                              n91 = Add(x=w258, y=w259) -> (x+y=w260:dbl)
                              n92 = Less Or Equal?(x=w260, y=6.0) -> (x <= y?=w262:bool)
                              n93 = case shown="False" w262 {
                                tunnel: [w265 w268] -> w263
                                tunnel: w257 -> [w264 w267]
                                frame False {
                                n94 = local read "DPT dif."() -> (w266:dbl)
                                n95 = Add(x=w264, y=w266) -> (x+y=w265:dbl)
                                }
                                frame True {
                                # "[15]"
                                n96 = local read "DPT dif."() -> (w269:dbl)
                                n97 = Add(x=w269, y="Incremento") -> (x+y=w270:dbl)
                                n98 = local write "DPT dif."(w270) -> ()
                                n99 = Add(x=w267, y=w270) -> (x+y=w268:dbl)
                                }
                              }
                            }
                            frame 2 {
                              # "[16]"
                              # "Se disminuye la potencia óptica"
                              n100 = local read "DPT dif."() -> (w277:dbl)
                              n101 = Add(x=w277, y=w273) -> (x+y=w274:dbl)
                              n102 = Greater Or Equal?(x=w274, y=-6.0) -> (x >= y?=w275:bool)
                              n103 = case shown="True" w275 {
                                tunnel: [w280 w284] -> w278
                                tunnel: w272 -> [w279 w283]
                                frame False {
                                n104 = local read "DPT dif."() -> (w281:dbl)
                                n105 = Add(x=w279, y=w281) -> (x+y=w280:dbl)
                                }
                                frame True {
                                # "[17]"
                                n106 = local read "DPT dif."() -> (w286:dbl)
                                n107 = local read "Incremento"() -> (w282:dbl)
                                n108 = Subtract(x=w286, y=w282) -> (x-y=w285:dbl)
                                n109 = local write "DPT dif."(w285) -> ()
                                n110 = Add(x=w283, y=w285) -> (x+y=w284:dbl)
                                }
                              }
                            }
                          }
                          n111 = Unbundle By Name(w239) -> ("Max Current A"=w238:dbl)
                          n112 = call "potencia a corriente.vi"("Max current A"=w238, "Potencia"=w241) -> ("Corriente"=w240:dbl)
                          n113 = local write "Potencia derecho"(w241) -> ()
                          n114 = To Word Integer(number=w240) -> (16bit integer=w246:i16)
                          n115 = Type Cast(x=w246) -> (*(type *) &x=w245:string)  [unwired: 1 in]
                          n116 = Concatenate Strings("Aw", w245) -> (w244:string)
                          "Command to Port" <- w244
                          n117 = call "write read Lens Driver.vi"("VISA resource name"=w251, "command"=w244, "Calibration"=w239, "error in (no error)"=w252) -> ("VISA resource name out"=w248:refnum<visa-resource-name>, "Calibration 2"=→"Calibration 2":T3, "OK"=→"OK":bool, "Data"=→"Data":string, "error out"=w253:errorcluster)  [unwired: 4 in, 3 out]
                          "VISA resource name out" <- w248
                        }
                      }
                      n118 = local read "Parar adquisicion"() -> (w222:bool)
                      n119 = local read "Distancia"() -> (w219:u32)
                      n120 = local read "Auto scale X"() -> (w220:u8)
                      n121 = Build Array (concatenate)(w218, w219) -> (w214:u32[])
                      n122 = local read "Auto scale Y"() -> (w221:u8)
                      n123 = Build Array (concatenate)(w217, w216) -> (w215:dbl[])
                      n124 = case shown="0, Default" w221 {
                        frame 0, Default {
                          n125 = local read "Escala Y max"() -> (w233:dbl)
                          n126 = local read "Escala Y min"() -> (w232:dbl)
                          n127 = property on="Potencia optica y distancia" class="WFChart (strict)"("YScale.Maximum"=w233) -> ()  [unwired: 2 in, 2 out]
                          n128 = property on="Potencia optica y distancia" class="WFChart (strict)"("YScale.Minimum"=w232) -> ()  [unwired: 2 in, 2 out]
                        }
                        frame 1 {
                        }
                      }
                      n129 = case shown="0, Default" w220 {
                        frame 0, Default {
                          n130 = local read "Escala X min"() -> (w230:dbl)
                          n131 = local read "Escala X max"() -> (w231:dbl)
                          n132 = property on="Potencia optica y distancia" class="WFChart (strict)"("XScale.Maximum"=w231) -> ()  [unwired: 2 in, 2 out]
                          n133 = property on="Potencia optica y distancia" class="WFChart (strict)"("XScale.Minimum"=w230) -> ()  [unwired: 2 in, 2 out]
                        }
                        frame 1 {
                        }
                      }
                      n134 = property on="Potencia optica y distancia" class="WFChart (strict)"("XScale.ScaleFit"=w220) -> ()  [unwired: 2 in, 2 out]
                      n135 = Build Array(w215, w214) -> (w213:dbl[][])
                      n136 = property on="Potencia optica y distancia" class="WFChart (strict)"("YScale.ScaleFit"=w221) -> ()  [unwired: 2 in, 2 out]
                      n137 = Transpose 2D Array(2D array=w213) -> (transposed array=w212:dbl[][])
                      n138 = local write "Potencia optica y distancia"(w212) -> ()
                    }
                  }
                  frame Error {
                  }
                }
                n139 = call-poly <vilib>:"DAQmx Timing.vi"("task/channels in"=w45, "sample mode"=w38, "rate"="Frecuencia muestreo", "error in"=w44) -> ("task out"=w43:refnum<k21>, "error out"=w42:errorcluster)  [unwired: 10 in]
                n140 = Obtain Queue(max queue size (-1, unlimited)=w97, element data type="Cola tipo") -> (queue out=w94:refnum<queue>, error out=w95:errorcluster)  [unwired: 3 in, 1 out]
                n141 = call <vilib>:"DAQmx Start Task.vi"("task/channels in"=w43, "error in"=w42) -> ("task out"=w102:refnum<k21>, "error out"=w101:errorcluster)  [unwired: 12 in]
                n142 = Enqueue Element(queue=w93, element=0.0) -> (queue out=w70:refnum<queue>)  [unwired: 2 in, 2 out]
                n143 = while {
                  stop <- w110 stop-if-true
                  n144 = local read "Modo de video"() -> (w106:u16)
                  n145 = local read "Calidad"() -> (w107:u32)
                  n146 = local read "Frame Rate"() -> (w108:u32)
                  n147 = local read "Parar adquisicion"() -> (w109:bool)
                  n148 = call "grabarVideoSinGuardar.vi"("VideoMode"=w106, "Quality"=w107, "Stop (F)"=w109, "Frame Rate"=w108) -> ("Image Out"=w105:T1, "Stopped"=w110:bool)  [unwired: 21 in, 1 out]
                  n149 = local write "Image Out"(w105) -> ()
                }
                n150 = while {
                  tunnel: w70 -> [w298]
                  tunnel: w94 -> [w315]
                  shift-right: [w301] -> _
                  shift-left: dbl[] [0.0] -> [w312]
                  shift-right: [w300] -> _
                  shift-left: u32[] [0] -> [w302]
                  tunnel: [w298] -> w68
                  stop <- w313 stop-if-true
                  # "[11]"
                  # "[10]"
                  # "[9]"
                  # "[8]"
                  # "[7]"
                  # "[6]"
                  n151 = local read "Parar adquisicion"() -> (w313:bool)
                  n152 = call "waveform_length.vi"("WL"="WL", "Cola WL"=w298, "Datos entrada"=w315) -> ("WL 2"=w310:dbl)
                  n153 = local write "WL"(w310) -> ()
                  n154 = Build Array (concatenate)(w312, w310) -> (w301:dbl[])
                  n155 = In Range and Coerce(upper limit="Limite superior WL", x=w310, lower limit="Limite inferior WL") -> (In Range?=w308:bool)  [unwired: 1 out]
                  n156 = Greater?(x=w310, y="Limite superior WL") -> (0:w309:bool)
                  n157 = Build Array(w309, w308) -> (w307:bool[])
                  n158 = Boolean Array To Number(Boolean array=w307) -> (number=w303:u32)
                  "number" <- w303
                  n159 = Build Array (concatenate)(w302, w303) -> (w300:u32[])
                  n160 = Build Array(w301, w300) -> (w299:dbl[][])
                  n161 = Transpose 2D Array(2D array=w299) -> (transposed array=→"Waveform length":dbl[][])
                  n162 = property on="Waveform length" class="WFChart (strict)"("YScale.ScaleFit"="Escala autom. Y") -> ()  [unwired: 2 in, 2 out]
                  n163 = property on="Waveform length" class="WFChart (strict)"("XScale.ScaleFit"="Escala autom. X") -> ()  [unwired: 2 in, 2 out]
                  n164 = case shown="0, Default" "Escala autom. Y" {
                    frame 0, Default {
                      n165 = property on="Waveform length" class="WFChart (strict)"("YScale.Maximum"="Maximo escala Y") -> ()  [unwired: 2 in, 2 out]
                      n166 = property on="Waveform length" class="WFChart (strict)"("YScale.Minimum"="Minimo escala Y") -> ()  [unwired: 2 in, 2 out]
                    }
                    frame 1 {
                    }
                  }
                  n167 = case shown="0, Default" "Escala autom. X" {
                    frame 0, Default {
                      n168 = property on="Waveform length" class="WFChart (strict)"("XScale.Minimum"="Minimo escala X") -> ()  [unwired: 2 in, 2 out]
                      n169 = property on="Waveform length" class="WFChart (strict)"("XScale.Maximum"="Maximo escala X") -> ()  [unwired: 2 in, 2 out]
                    }
                    frame 1 {
                    }
                  }
                }
                n170 = while {
                  tunnel: w102 -> [w341]
                  tunnel: "tamaño buffer" -> [w338]
                  tunnel: [w339] -> w98
                  shift-right: [w336] -> w99
                  shift-left: w101 -> [w340]
                  tunnel: [w330] -> _
                  tunnel: w94 -> [w326]
                  tunnel: w95 -> [w325]
                  stop <- w335 stop-if-true
                  w334 = 10.0  # timeout (s)
                  # "[5]"
                  # "[4]"
                  # "[3]"
                  # "[2]"
                  n171 = case shown="0, Default" "Escala automatica X" {
                    frame 0, Default {
                      n172 = property on="Senal EMG" class="WFGraph (strict)"("XScale.Increment"="X Scale.Range:Increment") -> ()  [unwired: 2 in, 2 out]
                      n173 = property on="Senal EMG" class="WFGraph (strict)"("XScale.Minimum"="X Scale.Range:Minimum") -> ()  [unwired: 2 in, 2 out]
                      n174 = property on="Senal EMG" class="WFGraph (strict)"("XScale.Maximum"="X Scale.Range:Maximum") -> ()  [unwired: 2 in, 2 out]
                    }
                    frame 1 {
                    }
                  }
                  n175 = call-poly <vilib>:"DAQmx Read.vi"("task/channels in"=w341, "number of samples per channel"=w338, "timeout"=w334, "error in"=w340) -> ("task out"=w339:refnum<k21>, "data"=w330:waveform(dbl)[], "error out"=w336:errorcluster)  [unwired: 9 in]
                  "Senal EMG" <- w330
                  n176 = call-poly <vilib>:"Index Waveform Array.vi"("index"=0, "waveform array"=w330) -> ("waveform"=w331:waveform(dbl))  [unwired: 8 in, 1 out]
                  n177 = Unbundle By Name(w331) -> ("Y"=w328:dbl[])  [unwired: 2 out]
                  n178 = local read "factor decimacion"() -> (w327:i32)
                  n179 = Unbundle By Name(w336) -> ("status"=w337:bool)
                  n180 = Or(x=w337, y="Parar adquisicion") -> (x .or. y?=w335:bool)
                  n181 = case shown="0, Default" "Escala automatica Y" {
                    frame 0, Default {
                      n182 = property on="Senal EMG" class="WFGraph (strict)"("YScale.Minimum"="Y Scale.Range:Minimum") -> ()  [unwired: 2 in, 2 out]
                      n183 = property on="Senal EMG" class="WFGraph (strict)"("YScale.Maximum"="Y Scale.Range:Maximum") -> ()  [unwired: 2 in, 2 out]
                    }
                    frame 1 {
                    }
                  }
                  n184 = call-poly <vilib>:"Decimate (continuous).vi"("averaging"=TRUE, "decimating factor"=w327, "X"=w328) -> ("Decimated Array"=w324:dbl[])  [unwired: 7 in, 1 out]
                  n185 = Lossy Enqueue Element(queue=w326, element=w324, error in (no error)=w325) -> ()  [unwired: 4 out]
                  n186 = property on="Senal EMG" class="WFGraph (strict)"("YScale.ScaleFit"="Escala automatica Y") -> ()  [unwired: 2 in, 2 out]
                  n187 = property on="Senal EMG" class="WFGraph (strict)"("XScale.ScaleFit"="Escala automatica X") -> ()  [unwired: 2 in, 2 out]
                  n188 = local read "Ganancia"() -> (w321:u16)
                  n189 = event shown="[0] \"Ganancia\": Value Change" {
                    selector: _ -> [_ _]
                    dyn-events: _ -> [_ _]
                    timeout: 10 -> [_ _]
                    tunnel: w321 -> [w342 _]
                    event "Ganancia": Value Change {
                      n190 = event-data() -> ()  [unwired: 1 in, 4 out]
                      n191 = call "Ganancia programable.vi"("MOSI data"=w342) -> ()
                    }
                    event Timeout {
                      n192 = event-data() -> ()  [unwired: 1 in, 3 out]
                    }
                  }
                }
                n193 = call <vilib>:"DAQmx Clear Task.vi"("task in"=w98, "error in"=w99) -> ()  [unwired: 13 in, 1 out]
                n194 = Flush Queue(queue=w68) -> ()  [unwired: 1 in, 3 out]
                n195 = VISA Close(VISA resource name=w47, error in (no error)=w46) -> (error out=w48:errorcluster)
                n196 = call <vilib>:"Simple Error Handler.vi"("error in (no error)"=w48) -> ("error out"=→"error out 2":errorcluster)  [unwired: 4 in, 4 out]
                n197 = VISA Close(VISA resource name=w74, error in (no error)=w76) -> (error out=w77:errorcluster)
                n198 = call <vilib>:"Simple Error Handler.vi"("error in (no error)"=w77) -> ("error out"=→"error out":errorcluster)  [unwired: 4 in, 4 out]
              }
              frame 2 {
                w368 = u16 0 items=["None", "Last Bit", "TermChar", "Break"] ("Serial Settings:End Mode for Writes")
                w367 = u16 2 items=["None", "Last Bit", "TermChar"] ("Serial Settings:End Mode for Reads")
                w381 = u16 0 items=["None", "Last Bit", "TermChar", "Break"] ("Serial Settings:End Mode for Writes")
                w380 = u16 2 items=["None", "Last Bit", "TermChar"] ("Serial Settings:End Mode for Reads")
                # "En esta opcion se configura la potencia inicial de los lentes"
                # "Close VISA port after program stop. Otherwise this port is blocked."
                # "Close VISA port after program stop. Otherwise this port is blocked."
                # "PwTA command to set temperature limits: PwTA as ASCII characters followed by 45 and 20 degrees in binary code."
                # "Initialize VISA port with correct parameters"
                # "PwTA command to set temperature limits: PwTA as ASCII characters followed by 45 and 20 degrees in binary code."
                # "Initialize VISA port with correct parameters"
                n199 = local read "VISA resource name"() -> (w358:string)
                n200 = call-poly "VISA Configure Serial Port"("VISA resource name"=w358, "timeout (10sec)"=u32 2000, "Enable Termination\nChar (T)"=FALSE ("Enable Termination\nChar (T)"), "baud rate (9600)"=u32 115200, "error in (no error)"="error in (no error) 3") -> ("VISA resource name out"=w363:refnum<visa-resource-name>, "error out"=w365:errorcluster)  [unwired: 9 in]
                n201 = property class="Instr"(reference=w363, error in=w365, "TermChar"=u8 10 ("Message Based Settings:Termination Character"), "ASRL End In"=w367, "ASRL End Out"=w368) -> (reference out=w364:refnum<visa-resource-name>, error out=w366:errorcluster)
                n202 = VISA Set I/O Buffer Size(VISA resource name=w364, error in (no error)=w366) -> (VISA resource name out=w370:refnum<visa-resource-name>, error out=w371:errorcluster)  [unwired: 2 in]
                n203 = VISA Flush I/O Buffer(VISA resource name=w370, error in (no error)=w371) -> (VISA resource name out=w357:refnum<visa-resource-name>, error out=w356:errorcluster)  [unwired: 1 in]
                n204 = case shown="No Error" w356 {
                  tunnel: w356 -> [w403 w437]
                  tunnel: w357 -> [w402 w438]
                  tunnel: [w401 w437] -> w352
                  tunnel: [w400 w438] -> w353
                  frame No Error {
                    w399 = 2 ("length (rest)")
                    # "Initialize Lens Driver"
                    n205 = local read "Calibration"() -> (w391:T3)
                    n206 = for {
                      tunnel: w402 -> [w435]
                      tunnel: [w432] -> w394
                      tunnel: string[] ["Start", "MwDA", "CrMA00", "CrMB00", "CrUA00", "CrUB00", "CrLA00", "CrLB00", "PwTA\u0002Ð\u0001@"] -> [w430] mode=indexing
                      tunnel: [w429] -> w393
                      shift-right: [w433] -> w395
                      shift-left: w391 -> [w434]
                      shift-right: [w431] -> w396
                      shift-left: w403 -> [w436]
                      n207 = call "write read Lens Driver.vi"("VISA resource name"=w435, "command"=w430, "Calibration"=w434, "error in (no error)"=w436) -> ("VISA resource name out"=w432:refnum<visa-resource-name>, "Calibration 2"=w433:T3, "Data"=w429:string, "error out"=w431:errorcluster)  [unwired: 4 in, 4 out]
                    }
                    n208 = String Subset(string=w393, offset (0)=w399, length (rest)=w399) -> (substring=w397:string)
                    n209 = Type Cast(type=u16 0 ("length (rest)"), x=w397) -> (*(type *) &x=w392:u16)
                    n210 = local write "ID"(w392) -> ()
                    n211 = while {
                      tunnel: [w405] -> w401
                      tunnel: [w406] -> w400
                      tunnel: w396 -> [w411]
                      tunnel: w395 -> [w410]
                      tunnel: w394 -> [w409]
                      stop <- w404 stop-if-true
                      # "When Send command is true, Current Ch A is sent to the Lens Driver, in the correct format. If answer exists it is displayed in Data. The update rate of the while loop is 2ms."
                      n212 = Wait Until Next ms Multiple(millisecond multiple=u32 2) -> ()  [unwired: 1 out]
                      n213 = case shown="True" TRUE ("Send command") {
                        tunnel: [w413 w428] -> w405
                        tunnel: w411 -> [w413 w427]
                        tunnel: w410 -> [_ w418]
                        tunnel: w409 -> [w412 w426]
                        tunnel: [w412 w419] -> w406
                        frame False {
                        }
                        frame True {
                          n214 = Unbundle By Name(w418) -> ("Max Current A"=w417:dbl)
                          n215 = call "potencia a corriente.vi"("Max current A"=w417, "Potencia"="Potencia inicial lente derecho") -> ("Corriente"=w415:dbl)
                          n216 = To Word Integer(number=w415) -> (16bit integer=w425:i16)
                          n217 = Type Cast(x=w425) -> (*(type *) &x=w424:string)  [unwired: 1 in]
                          n218 = Concatenate Strings("Aw", w424) -> (w421:string)
                          n219 = local write "Command to Port"(w421) -> ()
                          n220 = call "write read Lens Driver.vi"("VISA resource name"=w426, "command"=w421, "Calibration"=w418, "error in (no error)"=w427) -> ("VISA resource name out"=w419:refnum<visa-resource-name>, "Calibration 2"=w423:T3, "OK"=w422:bool, "Data"=w420:string, "error out"=w428:errorcluster)  [unwired: 4 in, 3 out]
                          n221 = local write "VISA resource name out"(w419) -> ()
                          n222 = local write "Calibration 2"(w423) -> ()
                          n223 = local write "Data"(w420) -> ()
                          n224 = local write "OK"(w422) -> ()
                          "DPT INICIALES D" <- "Potencia inicial lente derecho"
                        }
                      }
                      n225 = local read "Parar adquisicion"() -> (w404:bool)
                    }
                  }
                  frame Error {
                  }
                }
                n226 = VISA Close(VISA resource name=w353, error in (no error)=w352) -> (error out=w355:errorcluster)
                n227 = call <vilib>:"Simple Error Handler.vi"("error in (no error)"=w355) -> ("error out"=→"error out 3":errorcluster)  [unwired: 4 in, 4 out]
                n228 = local read "VISA resource name 2"() -> (w372:string)
                n229 = call-poly "VISA Configure Serial Port"("VISA resource name"=w372, "timeout (10sec)"=u32 2000, "Enable Termination\nChar (T)"=FALSE ("Enable Termination\nChar (T)"), "baud rate (9600)"=u32 115200, "error in (no error)"="error in (no error) 4") -> ("VISA resource name out"=w376:refnum<visa-resource-name>, "error out"=w378:errorcluster)  [unwired: 9 in]
                n230 = property class="Instr"(reference=w376, error in=w378, "TermChar"=u8 10 ("Message Based Settings:Termination Character"), "ASRL End In"=w380, "ASRL End Out"=w381) -> (reference out=w377:refnum<visa-resource-name>, error out=w379:errorcluster)
                n231 = VISA Set I/O Buffer Size(VISA resource name=w377, error in (no error)=w379) -> (VISA resource name out=w383:refnum<visa-resource-name>, error out=w384:errorcluster)  [unwired: 2 in]
                n232 = VISA Flush I/O Buffer(VISA resource name=w383, error in (no error)=w384) -> (VISA resource name out=w386:refnum<visa-resource-name>, error out=w385:errorcluster)  [unwired: 1 in]
                n233 = case shown="No Error" w385 {
                  tunnel: w385 -> [w452 w492]
                  tunnel: w386 -> [w451 w493]
                  tunnel: [w450 w492] -> w349
                  tunnel: [w449 w493] -> w348
                  frame No Error {
                    w448 = 2 ("length (rest)")
                    # "Initialize Lens Driver"
                    n234 = local read "Calibration"() -> (w440:T3)
                    n235 = for {
                      tunnel: w451 -> [w490]
                      tunnel: [w487] -> w443
                      tunnel: string[] ["Start", "MwDA", "CrMA00", "CrMB00", "CrUA00", "CrUB00", "CrLA00", "CrLB00", "PwTA\u0002Ð\u0001@"] -> [w485] mode=indexing
                      tunnel: [w484] -> w442
                      shift-right: [w488] -> w444
                      shift-left: w440 -> [w489]
                      shift-right: [w486] -> w445
                      shift-left: w452 -> [w491]
                      n236 = call "write read Lens Driver.vi"("VISA resource name"=w490, "command"=w485, "Calibration"=w489, "error in (no error)"=w491) -> ("VISA resource name out"=w487:refnum<visa-resource-name>, "Calibration 2"=w488:T3, "Data"=w484:string, "error out"=w486:errorcluster)  [unwired: 4 in, 4 out]
                    }
                    n237 = String Subset(string=w442, offset (0)=w448, length (rest)=w448) -> (substring=w446:string)
                    n238 = Type Cast(type=u16 0 ("length (rest)"), x=w446) -> (*(type *) &x=w441:u16)
                    n239 = local write "ID"(w441) -> ()
                    n240 = while {
                      tunnel: [w454] -> w450
                      tunnel: [w455] -> w449
                      tunnel: w445 -> [w460]
                      tunnel: w444 -> [w459]
                      tunnel: w443 -> [w458]
                      stop <- w453 stop-if-true
                      # "When Send command is true, Current Ch A is sent to the Lens Driver, in the correct format. If answer exists it is displayed in Data. The update rate of the while loop is 2ms."
                      n241 = Wait Until Next ms Multiple(millisecond multiple=u32 2) -> ()  [unwired: 1 out]
                      n242 = case shown="True" TRUE ("Send command") {
                        tunnel: [w462 w483] -> w454
                        tunnel: w460 -> [w462 w482]
                        tunnel: w459 -> [_ w470]
                        tunnel: w458 -> [w461 w481]
                        tunnel: [w461 w471] -> w455
                        frame False {
                        }
                        frame True {
                          n243 = Unbundle By Name(w470) -> ("Max Current A"=w469:dbl)
                          n244 = Multiply(x=15.8, y="Potencia inicial lente izquierdo") -> (x*y=w467:dbl)
                          n245 = Add(x=-6.8, y=w467) -> (x+y=w465:dbl)
                          n246 = Divide(x=w465, y=w469) -> (x/y=w468:dbl)
                          n247 = Multiply(x=4096.0, y=w468) -> (x*y=w479:dbl)
                          n248 = To Word Integer(number=w479) -> (16bit integer=w478:i16)
                          n249 = Type Cast(x=w478) -> (*(type *) &x=w477:string)  [unwired: 1 in]
                          n250 = Concatenate Strings("Aw", w477) -> (w473:string)
                          n251 = local write "Command to Port"(w473) -> ()
                          n252 = call "write read Lens Driver.vi"("VISA resource name"=w481, "command"=w473, "Calibration"=w470, "error in (no error)"=w482) -> ("VISA resource name out"=w471:refnum<visa-resource-name>, "Calibration 2"=w475:T3, "OK"=w474:bool, "Data"=w472:string, "error out"=w483:errorcluster)  [unwired: 4 in, 3 out]
                          n253 = local write "VISA resource name out 2"(w471) -> ()
                          n254 = local write "Calibration 2"(w475) -> ()
                          n255 = local write "Data"(w472) -> ()
                          n256 = local write "OK"(w474) -> ()
                          "DPT INICIALES I" <- "Potencia inicial lente izquierdo"
                        }
                      }
                      n257 = local read "Parar adquisicion"() -> (w453:bool)
                    }
                  }
                  frame Error {
                  }
                }
                n258 = VISA Close(VISA resource name=w348, error in (no error)=w349) -> (error out=w351:errorcluster)
                n259 = call <vilib>:"Simple Error Handler.vi"("error in (no error)"=w351) -> ("error out"=→"error out 4":errorcluster)  [unwired: 4 in, 4 out]
              }
              frame 1 {
                # "Mensaje que pregunta si desea realizar el experimento\ncon un nuevo usuario o con el actual"
                # "Se vuelven 0 los valores del WL y de la potencia óptica y distancia"
                # "En esta opcion se activa el modo experimento"
                n260 = property on="Waveform length" class="WFChart (strict)"("History Data"=dbl[][] [[0.0]]) -> ()  [unwired: 2 in, 2 out]
                n261 = property on="Potencia optica y distancia" class="WFChart (strict)"("History Data"=dbl[][] [[0.0]]) -> ()  [unwired: 2 in, 2 out]
                n262 = Two Button Dialog(message="Con quien desea realizar los experimentos?", 1:"Nuevo voluntario" ("F button name (\"Cancel\")"), 2:"Voluntario actual" ("T button name (\"OK\")")) -> (T button?=w512:bool)
                n263 = flat-sequence {
                  tunnel: w512 -> [w525]
                  tunnel: [w524] -> w510
                  tunnel: w509 -> [w524]
                  tunnel: [w517] -> w497
                  tunnel: w496 -> [w517]
                  tunnel: [w535] -> w513
                  tunnel: [w537] -> w511
                  tunnel: w510 -> [w537]
                  tunnel: [w536] -> w507
                  tunnel: w506 -> [w536]
                  tunnel: [w534] -> w498
                  tunnel: w497 -> [w534]
                  tunnel: w513 -> [w549]
                  tunnel: w511 -> [w548]
                  tunnel: [w547] -> w508
                  tunnel: w507 -> [w546]
                  tunnel: [w545] -> w504
                  tunnel: [w544] -> w503
                  tunnel: [w543] -> w501
                  tunnel: [w542] -> w499
                  tunnel: w498 -> [w542]
                  tunnel: w504 -> [w598]
                  tunnel: w503 -> [w581]
                  tunnel: [w598] -> w502
                  tunnel: w501 -> [w584]
                  tunnel: [w574] -> w500
                  tunnel: w499 -> [w574]
                  tunnel: [w601] -> w505
                  tunnel: w502 -> [w601]
                  tunnel: w500 -> [w599]
                  frame #0 {
                    # "Se guardan los datos de un nuevo voluntario"
                    n264 = Not(x=w525) -> (.not. x?=w519:bool)
                    n265 = case shown="True" w519 {
                      tunnel: [w528 w533] -> w523
                      tunnel: [w527 w532] -> w522
                      tunnel: [w529 w531] -> w521
                      tunnel: [w526 w530] -> w520
                      frame False {
                        n266 = local read "Enfermedad visual"() -> (w528:string)
                        n267 = local read "Nombre"() -> (w529:string)
                        n268 = local read "Cedula"() -> (w526:string)
                        n269 = local read "Edad"() -> (w527:string)
                      }
                      frame True {
                        n270 = call "Registro voluntario"() -> ("Enfermedad visual"=w533:string, "Edad"=w532:string, "Cedula"=w530:string, "Nombre"=w531:string)  [unwired: 14 in, 2 out]
                      }
                    }
                    "Cedula" <- w520
                    "Nombre" <- w521
                    "Edad" <- w522
                    "Enfermedad visual" <- w523
                    n271 = local write "T button?"(FALSE ("T button?")) -> ()
                  }
                  frame #1 {
                    n272 = Two Button Dialog(message="Qué tipo de experimento desea realizar?", 1:"Nuevo Experimento" ("F button name (\"Cancel\")"), 2:"Experimento existente" ("T button name (\"OK\")")) -> (T button?=w538:bool)
                    n273 = Not(x=w538) -> (.not. x?=w535:bool)
                  }
                  frame #2 {
                    # "A partir de la seleccion del experimento, se obtiene la descripcion correspondiente que será guardada en el archivo"
                    n274 = case shown="False" w549 {
                      tunnel: w548 -> [w551 w569]
                      tunnel: [w551 w568] -> w547
                      tunnel: w546 -> [w553 w567]
                      tunnel: [w553 w566] -> w545
                      tunnel: [w554 w565] -> w544
                      tunnel: [w550 w564] -> w543
                      frame False {
                        n275 = call "Display Message to User"() -> ()  [unwired: 10 in, 2 out]
                        n276 = flat-sequence {
                          tunnel: [w555] -> w552
                          tunnel: w551 -> [w555]
                          tunnel: [w563] -> w554
                          tunnel: w553 -> [w562]
                          tunnel: ["Menu experimentos"] -> _
                          tunnel: w552 -> [w560]
                          tunnel: [w559] -> w550
                          frame #0 {
                            n277 = while {
                              stop <- w556 stop-if-true
                              # "El sistema se queda en el loop hasta que el usuario elija el experimento que desea realizar"
                              n278 = event shown="[0] \"Elegir menu Exp\": Value Change" {
                                selector: _ -> [_ _]
                                dyn-events: _ -> [_ _]
                                timeout: _ -> [_ _]
                                tunnel: [TRUE FALSE] -> w556
                                event "Elegir menu Exp": Value Change {
                                n279 = event-data() -> ()  [unwired: 1 in, 4 out]
                                }
                                event Timeout {
                                n280 = event-data() -> ()  [unwired: 1 in, 3 out]
                                }
                              }
                            }
                          }
                          frame #1 {
                            n281 = Index Array(array=w562, index="Menu experimentos") -> (element=w563:string)
                            n282 = Index Array(array=w560, index="Menu experimentos") -> (element=w559:string)
                          }
                        }
                        "Array" <- w551
                      }
                      frame True {
                        # "Se añade el nuevo experimento al menu de seleccion de experimentos"
                        # "Se guarda el nuevo experimento en el archivo que los contiene"
                        n283 = call "Nuevo experimento"() -> ("Descripcion"=w565:string, "Nombre"=w564:string)  [unwired: 16 in, 2 out]
                        n284 = Insert Into Array(array=w567, new element=w565) -> (w566:string[])  [unwired: 1 in]
                        n285 = Insert Into Array(array=w569, new element=w564) -> (w568:string[])  [unwired: 1 in]
                        n286 = property on="Menu experimentos" class="Ring (strict)"("Strings []"=w568) -> ()  [unwired: 2 in, 2 out]
                        n287 = Insert Into Array(array=string[] [], new element #1=w564, new element #2=w565) -> (w571:string[])  [unwired: 1 in]
                        n288 = call-poly <vilib>:"Write Delimited Spreadsheet.vi"("file path (dialog if empty)"=path "C:/Users/TGM1603/Documents/LabVIEW Data/Experimentos_realizados", "1D data"=w571, "append to file? (new file:F)"=TRUE) -> ()  [unwired: 11 in, 2 out]
                      }
                    }
                  }
                  frame #3 {
                    # "Se guardan los datos generales del experimento en el archivo de excel"
                    n289 = local read "Frecuencia muestreo"() -> (w576:i32)
                    n290 = local read "factor decimacion"() -> (w580:i32)
                    n291 = local read "Enfermedad visual"() -> (w583:string)
                    n292 = local read "Cedula"() -> (w585:string)
                    n293 = local read "Edad"() -> (w582:string)
                    n294 = local read "Nombre"() -> (w586:string)
                    n295 = Get Date/Time In Seconds() -> (seconds since 1Jan1904=w597:timestamp)
                    n296 = Path To String(path="Carpeta") -> (string=w593:string)
                    n297 = Format Date/Time String(time format string (%c)="_%d-%m-%y_%H-%M", seconds (now)=w597) -> (date/time string=w595:string)  [unwired: 1 in]
                    n298 = Number To Fractional String(number=w580, precision (6)=i16 0) -> (F-format string=w579:string)  [unwired: 2 in]
                    n299 = local read "Cedula"() -> (w589:string)
                    n300 = Number To Fractional String(number=w576, precision (6)=i16 0) -> (F-format string=w577:string)  [unwired: 2 in]
                    n301 = Concatenate Strings(w593, "\\" ("string"), w589, w595, "_" ("string"), w584, ".xlsx" ("string")) -> (w591:string)
                    n302 = String To Path(string=w591) -> (path=w590:path)
                    "path" <- w590
                    n303 = call "MS Office Report"("Path to Save Report"=w590, "Cedula"=w585, "decimacion"=w579, "Edad"=w582, "Enfermedad"=w583, "Exp_nombre"=w584, "Experimento"=w581, "freq"=w577, "Nombre"=w586) -> ()  [unwired: 17 in, 2 out]
                    "Nombre 2" <- w584
                  }
                  frame #4 {
                    n304 = while {
                      shift-right: [w603] -> _
                      shift-left: enum16{"Inicio", "Tomar datos", ""}."Inicio" -> [w605]
                      tunnel: w599 -> [w602]
                      stop <- w604 stop-if-true
                      n305 = case shown="\"Tomar datos\"" w605 {
                        tunnel: [w606 w617] -> w603
                        tunnel: w602 -> [_ w612]
                        frame "Inicio", Default {
                          # "Se chequea si el usuario ha presionado el boton de comenzar el experimento. Si no lo ha hecho, se queda en este estado (0).\n Cuando lo presiona, pasa al estado de adquirir datios (1) ."
                          n306 = Select(t=enum16{"Inicio", "Tomar datos", ""}."Tomar datos", s="Iniciar experimento", f=enum16{"Inicio", "Tomar datos", ""}."Inicio") -> (s? t:f=w606:enum16{"Inicio", "Tomar datos", ""})
                        }
                        frame "Tomar datos" {
                          n307 = flat-sequence {
                            tunnel: [w710] -> w616
                            tunnel: [w709] -> w615
                            tunnel: [w708] -> w614
                            tunnel: [w707] -> w613
                            tunnel: w612 -> [w701]
                            tunnel: [w684] -> w611
                            tunnel: [w664] -> w610
                            tunnel: w616 -> [w1024]
                            tunnel: w615 -> [w1023]
                            tunnel: w614 -> [w1022]
                            tunnel: w613 -> [w1021]
                            tunnel: w611 -> [w1018]
                            tunnel: w610 -> [w1019]
                            tunnel: [enum16{"Inicio", "Tomar datos", ""}."Inicio"] -> w617
                            frame #0 {
                              w621 = 10123 items=["Finite Samples"=10178, "Continuous Samples"=10123, "Hardware Timed Single Point"=12522] ("sample mode")
                              w625 = 10083 items=["Default"=-1, "RSE"=10083, "NRSE"=10078, "Differential"=10106, "Pseudodifferential"=12529] ("input terminal configuration")
                              w650 = u16 0 items=["None", "Last Bit", "TermChar", "Break"] ("Serial Settings:End Mode for Writes")
                              w651 = u16 2 items=["None", "Last Bit", "TermChar"] ("Serial Settings:End Mode for Reads")
                              w675 = u16 0 items=["None", "Last Bit", "TermChar", "Break"] ("Serial Settings:End Mode for Writes")
                              w676 = u16 2 items=["None", "Last Bit", "TermChar"] ("Serial Settings:End Mode for Reads")
                              w699 = 100  # max queue size
                              # "[9] Se unen en una sola matriz los vectores de tiempo, distancia, potencia derecha y potencia izquierda."
                              # "[9]"
                              # "[12] Se unen en una sola matriz, los vectores de  tiempo de la señal EMG, amplitud de la señal EMG, tiempo de potencia óptica, distancia, potencia óptica derecha y potencia óptica izquierda, en ese orden."
                              # "[8]"
                              # "[7]"
                              # "[6]"
                              # "[5]"
                              # "Se usan registros de desplazamiento para concatenar en un solo vector los datos que se obtienen en cada iteracion. Así en \n[1] Se guarda la potencia del lente derecho.\n[2] Por medio de variables locales, se guarda la distancia que se obtuvo en el bloque de distancia.\n[3]  Por medio de variables locales, se guarda la potencia del lente izquierdo que se obtuvo en el bloque de control de potencia del lente izquierdo.\n[4] Se guarda el tiempo actual.\n[5] Se pasa el vector de de potencia derecha a variable a string con 2 cifras significativas. \n[6] Se ajusta el vector del tiempo para que se muestre un tiempo relativo, es decir, en donde el primer dato sea 0 y en los demas se aumente un dt.  Además, se pasa el vector a variable a string con 5 cifras significativas.\n[7] Se pasa el vector de de distancia a variable a string con 0 cifras significativas. \n[8] Se pasa el vector de de potencia izquierda a variable a string con 2 cifras significativas."
                              # "En esta cola se guarda los datos de la señal EMG\nEn el bloque de adquisición los añade al adquirirlos y  en el de procesamiento los elimina al procesarlos ."
                              # "Initialize VISA port with correct parameters"
                              # "Initialize VISA port with correct parameters"
                              # "Close VISA port after program stop. Otherwise this port is blocked."
                              # "Se adquiere la señal del circuito de adquisicion, en donde se define la frecuencia de muestreo y el factor de decimacion.\n[1] Se inicializa el canal de adquisicion\n[2] Se ajusta el canal para que lea muestras continuas y apartir de estas prooduzca waveform data.\n[3]  Se obtiene los datos de la señal: la amplitud Y, el tiempo de inicio y el delta t.\n[4] Se decima el vector de amplitud. \n[5] Se usan registros de desplazamiento para concatenenar en un solo vector los datos de la amplitud que se obtienen en cada iteración. \n[6] Se obtiene el vector del tiempo."
                              # "[11] Los vectores de amplitud y tiempo se transforman a formato texto con 4 y 5 cifras significativas respectivamente y se unen para formar un vector de 2 columnas."
                              # "[9] Se ajusta el vector del tiempo para que se muestre un tiempo relativo, es decir, en donde el primer dato sea 0 y en los demas se aumente un dt. \n[10] Se extrae el primer elemento del vector ya que este siempre es 0 y no aporta información"
                              # "[12]"
                              # "[11]"
                              # "[10]"
                              # "[9]"
                              # "[8] Se guarda la fecha/hora en que se inicio el experimento"
                              # "[7] Se usan registros de desplazamiento para concatenar en un solo vector los datos del tiempo que se obtienen en cada iteracion."
                              # "[1]"
                              n308 = while {
                                stop <- w738 stop-if-true
                                # "En este bloque se lleva a cabo la grabacion de video"
                                n309 = local read "Parar adquisicion"() -> (w733:bool)
                                n310 = call "grabarVideo.vi"("VideoMode"="Modo de video", "Quality"="Calidad", "Stop (F)"=w733, "Image Logging Path"="Carpeta archivo", "Frame Rate"="Frame Rate") -> ("Image Out"=→"Image Out":T1, "Stopped"=w738:bool)  [unwired: 20 in, 1 out]
                              }
                              n311 = local read "error in (no error)"() -> (w671:errorcluster)
                              n312 = local read "VISA resource name"() -> (w670:string)
                              n313 = local read "VISA resource name 2"() -> (w646:string)
                              n314 = call-poly "VISA Configure Serial Port"("VISA resource name"=w670, "timeout (10sec)"=u32 2000, "Enable Termination\nChar (T)"=FALSE ("Enable Termination\nChar (T)"), "baud rate (9600)"=u32 115200, "error in (no error)"=w671) -> ("VISA resource name out"=w680:refnum<visa-resource-name>, "error out"=w678:errorcluster)  [unwired: 9 in]
                              n315 = call-poly "VISA Configure Serial Port"("VISA resource name"=w646, "timeout (10sec)"=u32 2000, "Enable Termination\nChar (T)"=FALSE ("Enable Termination\nChar (T)"), "baud rate (9600)"=u32 115200, "error in (no error)"="error in (no error) 5") -> ("VISA resource name out"=w655:refnum<visa-resource-name>, "error out"=w653:errorcluster)  [unwired: 9 in]
                              n316 = property class="Instr"(reference=w680, error in=w678, "TermChar"=u8 10 ("Message Based Settings:Termination Character"), "ASRL End In"=w676, "ASRL End Out"=w675) -> (reference out=w679:refnum<visa-resource-name>, error out=w677:errorcluster)
                              n317 = property class="Instr"(reference=w655, error in=w653, "TermChar"=u8 10 ("Message Based Settings:Termination Character"), "ASRL End In"=w651, "ASRL End Out"=w650) -> (reference out=w654:refnum<visa-resource-name>, error out=w652:errorcluster)
                              n318 = VISA Set I/O Buffer Size(VISA resource name=w679, error in (no error)=w677) -> (VISA resource name out=w673:refnum<visa-resource-name>, error out=w672:errorcluster)  [unwired: 2 in]
                              n319 = VISA Set I/O Buffer Size(VISA resource name=w654, error in (no error)=w652) -> (VISA resource name out=w648:refnum<visa-resource-name>, error out=w647:errorcluster)  [unwired: 2 in]
                              n320 = VISA Flush I/O Buffer(VISA resource name=w673, error in (no error)=w672) -> (VISA resource name out=w669:refnum<visa-resource-name>, error out=w668:errorcluster)  [unwired: 1 in]
                              n321 = call-poly <vilib>:"DAQmx Create Virtual Channel.vi"("input terminal configuration"=w625, "physical channels"=tag "Dev1/ai0") -> ("task out"=w624:refnum<k21>, "error out"=w623:errorcluster)  [unwired: 12 in]
                              n322 = VISA Flush I/O Buffer(VISA resource name=w648, error in (no error)=w647) -> (VISA resource name out=w644:refnum<visa-resource-name>, error out=w643:errorcluster)  [unwired: 1 in]
                              n323 = invoke on="Parar adquisicion" class="Bool (strict)" method="Reinit To Default"() -> ()  [unwired: 3 in, 3 out]
                              n324 = Obtain Queue(max queue size (-1, unlimited)=w699, element data type="Cola tipo 2") -> (queue out=w698:refnum<queue>)  [unwired: 3 in, 2 out]
                              n325 = Enqueue Element(queue=w701, element=0.0) -> (queue out=w704:refnum<queue>)  [unwired: 2 in, 2 out]
                              n326 = call-poly <vilib>:"DAQmx Timing.vi"("task/channels in"=w624, "sample mode"=w621, "samples per channel"=1000, "rate"=1000.0, "error in"=w623) -> ("task out"=w619:refnum<k21>, "error out"=w618:errorcluster)  [unwired: 9 in]
                              n327 = call <vilib>:"DAQmx Start Task.vi"("task/channels in"=w619, "error in"=w618) -> ("task out"=w723:refnum<k21>, "error out"=w724:errorcluster)  [unwired: 12 in]
                              n328 = local read "tamaño buffer"() -> (w722:i32)
                              n329 = case shown="No Error" w643 {
                                tunnel: w643 -> [w754 w811]
                                tunnel: w644 -> [w753 w812]
                                tunnel: [w752 w811] -> w630
                                tunnel: [w751 w812] -> w629
                                tunnel: [w741 dbl[] [-30.0]] -> _
                                frame No Error {
                                w750 = 2 ("length (rest)")
                                # "Bloque de control del izquierdo. Se explica en el caso 0 de visualziación general"
                                # "Initialize Lens Driver"
                                n330 = local read "Calibration"() -> (w742:T3)
                                n331 = for {
                                tunnel: w753 -> [w808]
                                tunnel: [w805] -> w745
                                tunnel: string[] ["Start", "MwDA", "CrMA00", "CrMB00", "CrUA00", "CrUB00", "CrLA00", "CrLB00", "PwTA\u0002Ð\u0001@"] -> [w803] mode=indexing
                                tunnel: [w802] -> w744
                                shift-right: [w806] -> w746
                                shift-left: w742 -> [w807]
                                shift-right: [w804] -> w747
                                shift-left: w754 -> [w809]
                                n332 = call "write read Lens Driver.vi"("VISA resource name"=w808, "command"=w803, "Calibration"=w807, "error in (no error)"=w809) -> ("VISA resource name out"=w805:refnum<visa-resource-name>, "Calibration 2"=w806:T3, "Data"=w802:string, "error out"=w804:errorcluster)  [unwired: 4 in, 4 out]
                                }
                                n333 = String Subset(string=w744, offset (0)=w750, length (rest)=w750) -> (substring=w748:string)
                                n334 = Type Cast(type=u16 0 ("length (rest)"), x=w748) -> (*(type *) &x=w743:u16)
                                n335 = local write "ID"(w743) -> ()
                                n336 = while {
                                tunnel: [w759] -> w752
                                tunnel: [w760] -> w751
                                tunnel: w747 -> [w765]
                                tunnel: w746 -> [w764]
                                tunnel: w745 -> [w763]
                                shift-right: [w756] -> w741
                                shift-left: _ -> [w757]
                                stop <- w758 stop-if-true
                                # "When Send command is true, Current Ch A is sent to the Lens Driver, in the correct format. If answer exists it is displayed in Data. The update rate of the while loop is 2ms."
                                n337 = case shown="True" TRUE ("Send command") {
                                tunnel: [w771 w794] -> w759
                                tunnel: w765 -> [w771 w793]
                                tunnel: w764 -> [_ w774]
                                tunnel: w763 -> [w770 w792]
                                tunnel: [w770 w785] -> w760
                                tunnel: [dbl[] [-20.0] w784] -> w756
                                tunnel: w757 -> [_ w783]
                                frame False {
                                }
                                frame True {
                                n338 = local read "Potencia inicial lente izquierdo"() -> (w782:dbl)
                                n339 = local read "DPT dif."() -> (w781:dbl)
                                n340 = Add(x=w781, y=w782) -> (x+y=w777:dbl)
                                n341 = Absolute Value(x=w777) -> (abs(x)=w779:dbl)
                                n342 = Greater Or Equal?(x=6.0, y=w779) -> (x >= y?=w778:bool)
                                n343 = case shown="False" w778 {
                                tunnel: w777 -> [w797 w801]
                                tunnel: [w795 w801] -> w775
                                frame False {
                                n344 = Greater Or Equal?(x=u16 0, y=w797) -> (x >= y?=w798:bool)
                                n345 = case shown="False" w798 {
                                tunnel: [i16 6 ("x") i16 -6 ("x")] -> w795
                                frame False {
                                }
                                frame True {
                                }
                                }
                                }
                                frame True {
                                }
                                }
                                "Potencia izquierdo" <- w775
                                n346 = Unbundle By Name(w774) -> ("Max Current A"=w773:dbl)
                                n347 = call "potencia a corriente.vi"("Max current A"=w773, "Potencia"=w775) -> ("Corriente"=w776:dbl)
                                n348 = To Word Integer(number=w776) -> (16bit integer=w791:i16)
                                n349 = Type Cast(x=w791) -> (*(type *) &x=w790:string)  [unwired: 1 in]
                                n350 = Concatenate Strings("Aw", w790) -> (w787:string)
                                n351 = local write "Command to Port"(w787) -> ()
                                n352 = call "write read Lens Driver.vi"("VISA resource name"=w792, "command"=w787, "Calibration"=w774, "error in (no error)"=w793) -> ("VISA resource name out"=w785:refnum<visa-resource-name>, "Calibration 2"=w789:T3, "OK"=w788:bool, "Data"=w786:string, "error out"=w794:errorcluster)  [unwired: 4 in, 3 out]
                                n353 = local write "VISA resource name 2"(w785) -> ()
                                n354 = local write "Calibration 2"(w789) -> ()
                                n355 = local write "Data"(w786) -> ()
                                n356 = local write "OK"(w788) -> ()
                                n357 = Build Array (concatenate)(w783, w775) -> (w784:dbl[])
                                }
                                }
                                n358 = Wait Until Next ms Multiple(millisecond multiple=u32 10) -> ()  [unwired: 1 out]
                                n359 = local read "Parar adquisicion"() -> (w758:bool)
                                n360 = event shown="[0] \"Restablecer Iniciales\": Value Change" {
                                selector: _ -> [_ _]
                                dyn-events: _ -> [_ _]
                                timeout: 100 -> [_ _]
                                event "Restablecer Iniciales": Value Change {
                                n361 = event-data() -> ()  [unwired: 1 in, 3 out]
                                n362 = local read "Potencia inicial lente izquierdo"() -> (w766:dbl)
                                n363 = local read "Potencia inicial lente derecho"() -> (w767:dbl)
                                n364 = local write "Potencia izquierdo"(w766) -> ()
                                n365 = local write "Potencia derecho"(w767) -> ()
                                n366 = local write "DPT dif."(0.0 ("DPT dif.")) -> ()
                                }
                                event Timeout {
                                n367 = event-data() -> ()  [unwired: 1 in, 3 out]
                                }
                                }
                                }
                                }
                                frame Error {
                                }
                              }
                              n368 = case shown="No Error" w668 {
                                tunnel: w668 -> [w834 w930]
                                tunnel: w669 -> [w833 w931]
                                tunnel: [w832 w930] -> w696
                                tunnel: [w831 w931] -> w695
                                tunnel: [w820 dbl[] [-1.0]] -> w688
                                tunnel: [w819 dbl[] [-30.0]] -> w636
                                tunnel: [w818 u32[] [0]] -> w666
                                tunnel: [w816 dbl[] [-30.0]] -> w639
                                frame No Error {
                                w830 = 2 ("length (rest)")
                                # "Bloque de control del lente derecho. Se explica en el caso 0 de visualziación general"
                                # "Initialize Lens Driver"
                                n369 = local read "Calibration"() -> (w822:T3)
                                n370 = for {
                                tunnel: w833 -> [w924]
                                tunnel: [w921] -> w825
                                tunnel: string[] ["Start", "MwDA", "CrMA00", "CrMB00", "CrUA00", "CrUB00", "CrLA00", "CrLB00", "PwTA\u0002Ð\u0001@"] -> [w919] mode=indexing
                                tunnel: [w918] -> w824
                                shift-right: [w922] -> w826
                                shift-left: w822 -> [w923]
                                shift-right: [w920] -> w827
                                shift-left: w834 -> [w925]
                                n371 = call "write read Lens Driver.vi"("VISA resource name"=w924, "command"=w919, "Calibration"=w923, "error in (no error)"=w925) -> ("VISA resource name out"=w921:refnum<visa-resource-name>, "Calibration 2"=w922:T3, "Data"=w918:string, "error out"=w920:errorcluster)  [unwired: 4 in, 4 out]
                                }
                                n372 = String Subset(string=w824, offset (0)=w830, length (rest)=w830) -> (substring=w828:string)
                                n373 = Type Cast(type=u16 0 ("length (rest)"), x=w828) -> (*(type *) &x=w823:u16)
                                n374 = local write "ID"(w823) -> ()
                                n375 = while {
                                tunnel: [w852] -> w832
                                tunnel: [w853] -> w831
                                tunnel: w827 -> [w858]
                                tunnel: w826 -> [w857]
                                tunnel: w825 -> [w856]
                                shift-right: [w839] -> w820
                                shift-left: dbl[] [0.0] -> [w840]
                                shift-right: [w847] -> w819
                                shift-left: dbl[] [0.0] -> [w850]
                                shift-right: [w846] -> w818
                                shift-left: u32[] [0] -> [w849]
                                shift-right: [w837] -> w816
                                shift-left: dbl[] [0.0] -> [w836]
                                stop <- w851 stop-if-true
                                # "[4]"
                                # "[3]"
                                # "[2]"
                                # "When Send command is true, Current Ch A is sent to the Lens Driver, in the correct format. If answer exists it is displayed in Data. The update rate of the while loop is 2ms."
                                n376 = Wait Until Next ms Multiple(millisecond multiple=u32 10) -> ()  [unwired: 1 out]
                                n377 = case shown="True" TRUE ("Send command") {
                                tunnel: [w865 w884] -> w852
                                tunnel: w858 -> [w865 w883]
                                tunnel: w857 -> [_ w868]
                                tunnel: w856 -> [w864 w882]
                                tunnel: [w864 w874] -> w853
                                tunnel: [dbl[] [-20.0] w873] -> w847
                                tunnel: w850 -> [_ w872]
                                frame False {
                                }
                                frame True {
                                # "[1]"
                                n378 = local read "number"() -> (w879:u32)
                                n379 = local read "Potencia inicial lente derecho"() -> (w871:dbl)
                                n380 = case shown="2" w879 {
                                tunnel: [w885 w894 w909] -> w870
                                tunnel: w871 -> [w887 w889 w904]
                                tunnel: w871 -> [_ w888 w903]
                                frame 0, Default {
                                n381 = local read "DPT dif."() -> (w886:dbl)
                                n382 = Add(x=w887, y=w886) -> (x+y=w885:dbl)
                                }
                                frame 1 {
                                n383 = local read "DPT dif."() -> (w890:dbl)
                                n384 = Add(x=w889, y=w890) -> (x+y=w891:dbl)
                                n385 = Less Or Equal?(x=w891, y=6.0) -> (x <= y?=w893:bool)
                                n386 = case shown="True" w893 {
                                tunnel: [w896 w900] -> w894
                                tunnel: w888 -> [w895 w899]
                                frame False {
                                n387 = local read "DPT dif."() -> (w897:dbl)
                                n388 = Add(x=w895, y=w897) -> (x+y=w896:dbl)
                                }
                                frame True {
                                n389 = local read "DPT dif."() -> (w901:dbl)
                                n390 = local read "Incremento"() -> (w898:dbl)
                                n391 = Add(x=w901, y=w898) -> (x+y=w902:dbl)
                                n392 = local write "DPT dif."(w902) -> ()
                                n393 = Add(x=w899, y=w902) -> (x+y=w900:dbl)
                                }
                                }
                                }
                                frame 2 {
                                n394 = local read "DPT dif."() -> (w908:dbl)
                                n395 = Add(x=w908, y=w904) -> (x+y=w905:dbl)
                                n396 = Greater Or Equal?(x=w905, y=-6.0) -> (x >= y?=w906:bool)
                                n397 = case shown="True" w906 {
                                tunnel: [w911 w915] -> w909
                                tunnel: w903 -> [w910 w914]
                                frame False {
                                n398 = local read "DPT dif."() -> (w912:dbl)
                                n399 = Add(x=w910, y=w912) -> (x+y=w911:dbl)
                                }
                                frame True {
                                n400 = local read "DPT dif."() -> (w917:dbl)
                                n401 = local read "Incremento"() -> (w913:dbl)
                                n402 = Subtract(x=w917, y=w913) -> (x-y=w916:dbl)
                                n403 = local write "DPT dif."(w916) -> ()
                                n404 = Add(x=w914, y=w916) -> (x+y=w915:dbl)
                                }
                                }
                                }
                                }
                                "Potencia derecho" <- w870
                                n405 = Unbundle By Name(w868) -> ("Max Current A"=w867:dbl)
                                n406 = call "potencia a corriente.vi"("Max current A"=w867, "Potencia"=w870) -> ("Corriente"=w869:dbl)
                                n407 = To Word Integer(number=w869) -> (16bit integer=w881:i16)
                                n408 = Type Cast(x=w881) -> (*(type *) &x=w880:string)  [unwired: 1 in]
                                n409 = Concatenate Strings("Aw", w880) -> (w876:string)
                                n410 = local write "Command to Port"(w876) -> ()
                                n411 = call "write read Lens Driver.vi"("VISA resource name"=w882, "command"=w876, "Calibration"=w868, "error in (no error)"=w883) -> ("VISA resource name out"=w874:refnum<visa-resource-name>, "Calibration 2"=w878:T3, "OK"=w877:bool, "Data"=w875:string, "error out"=w884:errorcluster)  [unwired: 4 in, 3 out]
                                n412 = local write "VISA resource name out"(w874) -> ()
                                n413 = local write "Calibration 2"(w878) -> ()
                                n414 = local write "Data"(w875) -> ()
                                n415 = local write "OK"(w877) -> ()
                                n416 = Build Array (concatenate)(w872, w870) -> (w873:dbl[])
                                }
                                }
                                n417 = local read "Parar adquisicion"() -> (w851:bool)
                                n418 = local read "Potencia izquierdo"() -> (w835:dbl)
                                n419 = local read "Distancia"() -> (w848:u32)
                                n420 = property on="Potencia optica y distancia" class="WFChart (strict)"("YScale.ScaleFit"="Auto scale Y") -> ()  [unwired: 2 in, 2 out]
                                n421 = Get Date/Time In Seconds() -> (seconds since 1Jan1904=w841:timestamp)
                                n422 = To Double Precision Float(number=w841) -> (double precision float=w838:dbl)
                                n423 = property on="Potencia optica y distancia" class="WFChart (strict)"("XScale.ScaleFit"="Auto scale X") -> ()  [unwired: 2 in, 2 out]
                                n424 = Build Array (concatenate)(w840, w838) -> (w839:dbl[])
                                n425 = case shown="0, Default" "Auto scale Y" {
                                frame 0, Default {
                                n426 = property on="Potencia optica y distancia" class="WFChart (strict)"("YScale.Maximum"="Escala Y max") -> ()  [unwired: 2 in, 2 out]
                                n427 = property on="Potencia optica y distancia" class="WFChart (strict)"("YScale.Minimum"="Escala Y min") -> ()  [unwired: 2 in, 2 out]
                                }
                                frame 1 {
                                }
                                }
                                n428 = Build Array (concatenate)(w836, w835) -> (w837:dbl[])
                                n429 = Build Array (concatenate)(w849, w848) -> (w846:u32[])
                                n430 = case shown="0, Default" "Auto scale X" {
                                frame 0, Default {
                                n431 = property on="Potencia optica y distancia" class="WFChart (strict)"("XScale.Maximum"="Escala X max") -> ()  [unwired: 2 in, 2 out]
                                n432 = property on="Potencia optica y distancia" class="WFChart (strict)"("XScale.Minimum"="Escala X min") -> ()  [unwired: 2 in, 2 out]
                                }
                                frame 1 {
                                }
                                }
                                n433 = Build Array(w847, w846) -> (w845:dbl[][])
                                n434 = Transpose 2D Array(2D array=w845) -> (transposed array=→"Potencia optica y distancia":dbl[][])
                                }
                                }
                                frame Error {
                                }
                              }
                              n435 = while {
                                tunnel: w704 -> [w963]
                                shift-right: [w965] -> _
                                shift-left: dbl[] [0.0] -> [w971]
                                shift-right: [w964] -> _
                                shift-left: u32[] [0] -> [w966]
                                tunnel: [w963] -> w702
                                tunnel: w698 -> [w955]
                                stop <- w954 stop-if-true
                                # "Bloque de procesamiento.  Se explica en el caso 0 de visualización general"
                                n436 = local read "WL"() -> (w962:dbl)
                                n437 = local read "Parar adquisicion"() -> (w954:bool)
                                n438 = local read "Limite superior WL"() -> (w959:dbl)
                                n439 = call "waveform_length.vi"("WL"=w962, "Cola WL"=w963, "Datos entrada"=w955) -> ("WL 2"=w970:dbl)
                                n440 = local read "Limite inferior WL"() -> (w961:dbl)
                                n441 = local write "WL"(w970) -> ()
                                n442 = Build Array (concatenate)(w971, w970) -> (w965:dbl[])
                                n443 = In Range and Coerce(upper limit=w959, x=w970, lower limit=w961) -> (In Range?=w968:bool)  [unwired: 1 out]
                                n444 = Greater?(x=w970, y=w959) -> (0:w969:bool)
                                n445 = local read "Escala autom. X"() -> (w956:u8)
                                n446 = local read "Escala autom. Y"() -> (w957:u8)
                                n447 = Build Array(w969, w968) -> (w967:bool[])
                                n448 = Boolean Array To Number(Boolean array=w967) -> (number=w960:u32)
                                n449 = local write "number"(w960) -> ()
                                n450 = Build Array (concatenate)(w966, w960) -> (w964:u32[])
                                n451 = Build Array(w965, w964) -> (w958:dbl[][])
                                n452 = Transpose 2D Array(2D array=w958) -> (transposed array=w953:dbl[][])
                                n453 = local write "Waveform length"(w953) -> ()
                                n454 = property on="Waveform length" class="WFChart (strict)"("XScale.ScaleFit"=w956) -> ()  [unwired: 2 in, 2 out]
                                n455 = property on="Waveform length" class="WFChart (strict)"("YScale.ScaleFit"=w957) -> ()  [unwired: 2 in, 2 out]
                                n456 = case shown="0, Default" w957 {
                                frame 0, Default {
                                n457 = local read "Maximo escala Y"() -> (w975:dbl)
                                n458 = local read "Minimo escala Y"() -> (w974:dbl)
                                n459 = property on="Waveform length" class="WFChart (strict)"("YScale.Maximum"=w975) -> ()  [unwired: 2 in, 2 out]
                                n460 = property on="Waveform length" class="WFChart (strict)"("YScale.Minimum"=w974) -> ()  [unwired: 2 in, 2 out]
                                }
                                frame 1 {
                                }
                                }
                                n461 = case shown="0, Default" w956 {
                                frame 0, Default {
                                n462 = local read "Minimo escala X"() -> (w973:dbl)
                                n463 = local read "Maximo escala X"() -> (w972:dbl)
                                n464 = property on="Waveform length" class="WFChart (strict)"("XScale.Minimum"=w973) -> ()  [unwired: 2 in, 2 out]
                                n465 = property on="Waveform length" class="WFChart (strict)"("XScale.Maximum"=w972) -> ()  [unwired: 2 in, 2 out]
                                }
                                frame 1 {
                                }
                                }
                              }
                              n466 = while {
                                tunnel: w723 -> [w1008]
                                tunnel: w722 -> [w1005]
                                tunnel: [w1006] -> w712
                                shift-right: [w1003] -> w711
                                shift-left: w724 -> [w1007]
                                tunnel: [w998] -> w732
                                shift-right: [w997] -> w709
                                shift-left: _ -> [w996]
                                shift-right: [w987] -> w714
                                shift-left: dbl[] [0.0] -> [w992]
                                shift-right: [w988] -> w719
                                shift-left: dbl[] [0.0] -> [w989]
                                tunnel: w698 -> [w980]
                                i -> [w999]
                                stop <- w1002 stop-if-true
                                w1001 = 10.0  # timeout (s)
                                # "[7]"
                                # "[6]"
                                # "[5]"
                                # "[4]"
                                # "[3]"
                                # "[2]"
                                n467 = local read "Escala automatica X"() -> (w978:u8)
                                n468 = local read "Escala automatica Y"() -> (w977:u8)
                                n469 = property on="Senal EMG" class="WFGraph (strict)"("XScale.ScaleFit"=w978) -> ()  [unwired: 2 in, 2 out]
                                n470 = case shown="0, Default" w978 {
                                frame 0, Default {
                                n471 = local read "X Scale.Range:Increment"() -> (w1011:dbl)
                                n472 = local read "X Scale.Range:Minimum"() -> (w1012:dbl)
                                n473 = local read "X Scale.Range:Maximum"() -> (w1013:dbl)
                                n474 = property on="Senal EMG" class="WFGraph (strict)"("XScale.Increment"=w1011) -> ()  [unwired: 2 in, 2 out]
                                n475 = property on="Senal EMG" class="WFGraph (strict)"("XScale.Minimum"=w1012) -> ()  [unwired: 2 in, 2 out]
                                n476 = property on="Senal EMG" class="WFGraph (strict)"("XScale.Maximum"=w1013) -> ()  [unwired: 2 in, 2 out]
                                }
                                frame 1 {
                                }
                                }
                                n477 = local read "Parar adquisicion"() -> (w983:bool)
                                n478 = call-poly <vilib>:"DAQmx Read.vi"("task/channels in"=w1008, "number of samples per channel"=w1005, "timeout"=w1001, "error in"=w1007) -> ("task out"=w1006:refnum<k21>, "data"=w993:waveform(dbl)[], "error out"=w1003:errorcluster)  [unwired: 9 in]
                                n479 = Unbundle By Name(w1003) -> ("status"=w1004:bool)
                                n480 = Or(x=w1004, y=w983) -> (x .or. y?=w1002:bool)
                                n481 = property on="Senal EMG" class="WFGraph (strict)"("YScale.ScaleFit"=w977) -> ()  [unwired: 2 in, 2 out]
                                n482 = local write "Senal EMG"(w993) -> ()
                                n483 = case shown="0, Default" w977 {
                                frame 0, Default {
                                n484 = local read "Y Scale.Range:Maximum"() -> (w1010:dbl)
                                n485 = local read "Y Scale.Range:Minimum"() -> (w1009:dbl)
                                n486 = property on="Senal EMG" class="WFGraph (strict)"("YScale.Minimum"=w1009) -> ()  [unwired: 2 in, 2 out]
                                n487 = property on="Senal EMG" class="WFGraph (strict)"("YScale.Maximum"=w1010) -> ()  [unwired: 2 in, 2 out]
                                }
                                frame 1 {
                                }
                                }
                                n488 = call-poly <vilib>:"Index Waveform Array.vi"("index"=0, "waveform array"=w993) -> ("waveform"=w991:waveform(dbl))  [unwired: 8 in, 1 out]
                                n489 = Unbundle By Name(w991) -> ("Y"=w981:dbl[], "t0"=w998:timestamp)  [unwired: 1 out]
                                n490 = call-poly <vilib>:"Decimate (continuous).vi"("averaging"=TRUE, "decimating factor"="factor decimacion", "X"=w981) -> ("Decimated Array"=w976:dbl[])  [unwired: 7 in, 1 out]
                                n491 = Lossy Enqueue Element(queue=w980, element=w976) -> ()  [unwired: 1 in, 4 out]
                                n492 = Build Array (concatenate)(w992, w976) -> (w987:dbl[])
                                n493 = case shown="1" w999 {
                                tunnel: w998 -> [_ w1017]
                                tunnel: [w1015 w1016] -> w997
                                tunnel: w996 -> [w1015 _]
                                frame 0, Default {
                                }
                                frame 1 {
                                # "[8]"
                                n494 = Format Date/Time String(seconds (now)=w1017) -> (date/time string=w1016:string)  [unwired: 2 in]
                                }
                                }
                                n495 = local read "factor decimacion"() -> (w984:i32)
                                n496 = call-poly <vilib>:"Get Waveform Time Array.vi"("waveform in"=w991) -> ("X array"=w990:timestamp[])  [unwired: 9 in, 1 out]
                                n497 = event shown="[0] \"Ganancia\": Value Change" {
                                selector: _ -> [_ _]
                                dyn-events: _ -> [_ _]
                                timeout: 1 -> [_ _]
                                tunnel: "Ganancia" -> [w1014 _]
                                event "Ganancia": Value Change {
                                n498 = event-data() -> ()  [unwired: 1 in, 4 out]
                                n499 = call "Ganancia programable.vi"("MOSI data"=w1014) -> ()
                                }
                                event Timeout {
                                n500 = event-data() -> ()  [unwired: 1 in, 3 out]
                                }
                                }
                                n501 = To Double Precision Float(number=w990) -> (double precision float=w986:dbl[])
                                n502 = call-poly <vilib>:"Decimate (single shot).vi"("decimating factor"=w984, "X"=w986) -> ("Decimated Array"=w985:dbl[])  [unwired: 8 in, 1 out]
                                n503 = Build Array (concatenate)(w989, w985) -> (w988:dbl[])
                              }
                              n504 = call <vilib>:"DAQmx Clear Task.vi"("task in"=w712, "error in"=w711) -> ()  [unwired: 13 in, 1 out]
                              n505 = Index Array(array=w719, index=1) -> (element=w718:dbl)
                              n506 = Flush Queue(queue=w702) -> ()  [unwired: 1 in, 3 out]
                              n507 = Subtract(x=w719, y=w718) -> (x-y=w716:dbl[])
                              n508 = Delete From Array(array=w714, index=0) -> (array with subset deleted=w727:dbl[])  [unwired: 1 in, 1 out]
                              n509 = while {
                                shift-right: [w932] -> _
                                shift-left: _ -> [w933]
                                stop <- w937 stop-if-true
                                # "Este bloque adquiere la distancia (se explica en el caso 0 (visualizacion general)"
                                n510 = call "meididor de distancia archivo adicional.vi"() -> ("error out"=w940:errorcluster, "task out"=w941:refnum<k21>)  [unwired: 10 in]
                                n511 = call "DAQ Assistant2"("timeout (s)"=0.05) -> ("data"=w950:dynamicdata, "error out"=w938:errorcluster)  [unwired: 16 in, 1 out]
                                n512 = call <vilib>:"DAQmx Start Task.vi"("task/channels in"=w941, "error in"=w940) -> ("task out"=w944:refnum<k21>, "error out"=w945:errorcluster)  [unwired: 12 in]
                                n513 = call <vilib>:"DAQmx Is Task Done.vi"("task/channels in"=w944, "error in"=w945) -> ("task out"=w942:refnum<k21>, "error out"=w943:errorcluster)  [unwired: 11 in, 1 out]
                                n514 = Wait (ms)(milliseconds to wait=u32 200) -> ()  [unwired: 1 out]
                                n515 = call <vilib>:"Clear Errors.vi"("error in (no error)"=w938) -> ()  [unwired: 5 in, 2 out]
                                n516 = local read "Parar adquisicion"() -> (w937:bool)
                                n517 = call <vilib>:"DAQmx Clear Task.vi"("task in"=w942, "error in"=w943) -> ()  [unwired: 13 in, 1 out]
                                n518 = Multiply(x=1000000.0, y=w950) -> (x*y=w948:dynamicdata)
                                n519 = Divide(x=w948, y=58.0) -> (x/y=w934:dynamicdata)
                                n520 = Equal?(x=w934, y=0.0) -> (x = y?=w936:dynamicdata)
                                n521 = case shown="True" w936 {
                                tunnel: [w951 w952] -> w932
                                tunnel: w934 -> [w951 _]
                                tunnel: w933 -> [_ w952]
                                frame False {
                                }
                                frame True {
                                }
                                }
                                n522 = local write "Distancia"(w932) -> ()
                              }
                              n523 = Delete From Array(array=w716, index=0) -> (array with subset deleted=w726:dbl[])  [unwired: 1 in, 1 out]
                              n524 = local read "path"() -> (w710:path)
                              n525 = Format Date/Time String(seconds (now)=w732) -> (date/time string=w708:string)  [unwired: 2 in]
                              n526 = Number To Fractional String(use system decimal point (T)=FALSE, number=w727, precision (6)=i16 4) -> (F-format string=w662:string[])  [unwired: 1 in]
                              n527 = Number To Fractional String(use system decimal point (T)=FALSE, number=w726, precision (6)=i16 5) -> (F-format string=w663:string[])  [unwired: 1 in]
                              n528 = Build Array(w663, w662) -> (w725:string[][])
                              n529 = Transpose 2D Array(2D array=w725) -> (transposed array=w707:string[][])
                              n530 = Delete From Array(array=w636, index=0) -> (array with subset deleted=w635:dbl[])  [unwired: 1 in, 1 out]
                              n531 = Delete From Array(array=w666, index=0) -> (array with subset deleted=w632:u32[])  [unwired: 1 in, 1 out]
                              n532 = Index Array(array=w688, index=1) -> (element=w693:dbl)
                              n533 = Delete From Array(array=w639, index=0) -> (array with subset deleted=w638:dbl[])  [unwired: 1 in, 1 out]
                              n534 = VISA Close(VISA resource name=w629, error in (no error)=w630) -> (error out=w628:errorcluster)
                              n535 = Subtract(x=w688, y=w693) -> (x-y=w687:dbl[])
                              n536 = Number To Fractional String(use system decimal point (T)=FALSE, number=w635, precision (6)=i16 2) -> (F-format string=w659:string[])  [unwired: 1 in]
                              n537 = VISA Close(VISA resource name=w695, error in (no error)=w696) -> (error out=w697:errorcluster)
                              n538 = call <vilib>:"Simple Error Handler.vi"("error in (no error)"=w628) -> ("error out"=w627:errorcluster)  [unwired: 4 in, 4 out]
                              n539 = Number To Fractional String(number=w632, precision (6)=i16 0) -> (F-format string=w660:string[])  [unwired: 2 in]
                              n540 = Delete From Array(array=w687, index=0) -> (array with subset deleted=w692:dbl[])  [unwired: 1 in, 1 out]
                              n541 = call <vilib>:"Simple Error Handler.vi"("error in (no error)"=w697) -> ("error out"=w694:errorcluster)  [unwired: 4 in, 4 out]
                              n542 = Number To Fractional String(use system decimal point (T)=FALSE, number=w638, precision (6)=i16 2) -> (F-format string=w640:string[])  [unwired: 1 in]
                              n543 = local write "error out"(w694) -> ()
                              n544 = local write "error out"(w627) -> ()
                              n545 = Number To Fractional String(use system decimal point (T)=FALSE, number=w692, precision (6)=i16 5) -> (F-format string=w661:string[])  [unwired: 1 in]
                              n546 = Build Array(w663, w662, w661, w660, w659, w640) -> (w633:string[][])
                              n547 = Transpose 2D Array(2D array=w633) -> (transposed array=w664:string[][])
                              n548 = Build Array(w661, w660, w659, w640) -> (w684:string[][])
                            }
                            frame #1 {
                              # "[13]"
                              # "[13] En esta case structure, se decide que datos se van a guardar. Esto lo hace el SUBVI llamado guardar datos de amplitud y tiempo."
                              n549 = Transpose 2D Array(2D array=w1018) -> (transposed array=w1020:string[][])
                              n550 = call <vilib>:"Three Button Dialog.vi"("Right Button Text (\"Cancel\")"="Señal EMG, potencia optica y distancia" ("Right Button Text (\"Cancel\")"), "Center Button Text (\"No\")"="Potencia optica y distancia" ("Center Button Text (\"No\")"), "Left Button Text (\"Yes\")"="Señal EMG" ("Left Button Text (\"Yes\")"), "message"="Elija que datos desea guardar") -> ("Which Button?"=w1025:T4)  [unwired: 7 in]
                              n551 = case shown="\"Center Button\"" w1025 {
                                tunnel: w1024 -> [w1034 w1039 w1042]
                                tunnel: w1023 -> [w1033 w1038 w1043]
                                tunnel: w1022 -> [w1032 w1037 w1044]
                                tunnel: w1021 -> [w1031 _ _]
                                tunnel: w1020 -> [_ w1036 _]
                                tunnel: w1019 -> [_ _ w1040]
                                frame "Left Button", Default {
                                # "Se guarda solo la señal EMG y su tiempo de adquisición."
                                n552 = call "Guardar datos de Amplitud y Tiempo.vi"("path"=w1034, "Hora inicio"=w1033, "Hora fin"=w1032, "Datos experimento"=w1031, "column headers"=string[] ["Tiempo(s)", "Amplitud(V)"]) -> ()  [unwired: 1 in]
                                }
                                frame "Center Button" {
                                # "Se guarda la potenica del lente derecho, del lente izquierdo, la distancia y el tiempo de estas variables."
                                n553 = call "Guardar datos de Amplitud y Tiempo.vi"("path"=w1039, "Hora inicio"=w1038, "Hora fin"=w1037, "Datos experimento"=w1036, "column headers"=string[] ["Tiempo(s)", "Distancia (cm)", "Potencia Optica derecho", "Potencia optica izquierdo"]) -> ()  [unwired: 1 in]
                                }
                                frame "Right Button" {
                                # "Se guarda el tiempo de adquisición así como la amplitud de la señal EMG,  la potenica del lente derecho, del lente izquierdo, la distancia y el tiempo de estas variables."
                                n554 = call "Guardar datos de Amplitud y Tiempo.vi"("path"=w1042, "Hora inicio"=w1043, "Hora fin"=w1044, "Datos experimento"=w1040, "column headers"=string[] ["Tiempo EMG(s)", "Amplitud(V)", "Tiempo DPT(s)", "Distancia (cm)", "Potencia optica derecho", "Potencia optica izquierdo"]) -> ()  [unwired: 1 in]
                                }
                              }
                            }
                            frame #2 {
                              # "Si el usuario desea repetir el experimento se vuelve al estado inicio en donde se espera que comience el experimento. De lo contrario se sale del loop y vuelve al menu principal."
                              n555 = Two Button Dialog(message="¿Desea repetir el experimento?", 1:"No" ("F button name (\"Cancel\")"), 2:"Si" ("T button name (\"OK\")")) -> (T button?=w1047:bool)
                              n556 = Not(x=w1047) -> (.not. x?=→"T button?":bool)
                            }
                          }
                        }
                      }
                      n557 = local read "T button?"() -> (w604:bool)
                    }
                  }
                }
                "Array 2" <- w509
              }
            }
          }
          event Timeout {
            n558 = event-data() -> ()  [unwired: 1 in, 3 out]
          }
        }
        "Array 3" <- w31
      }
      "Array 4" <- w22
    }
  }
